vi "SIAM_test_Standalone-ZMQ-Dev.vi"() -> ()   [LabVIEW 2011]
doc: "Tool for TILL ID SIAM hardware test."
uses:
  SIAM_command.ctl
  SIAM-axis.ctl
  Christian/ZeroMQ/Neuer Ordner/File Group 0/vi.lib/addons/zeromq/zmq_socket.lvclass
  Christian/ZeroMQ/Neuer Ordner/File Group 0/vi.lib/addons/zeromq/socket_type.ctl
  Christian/ZeroMQ/Neuer Ordner/File Group 0/vi.lib/addons/zeromq/socket_options.ctl
  Christian/ZeroMQ/Neuer Ordner/File Group 0/vi.lib/addons/zeromq/zmq_context.lvclass
  Christian/ZeroMQ/Neuer Ordner/File Group 0/vi.lib/addons/zeromq/zeromq.lvlib
panel:
  in  "Stop":bool
  in  "recieve socket":refnum<class "zmq_socket.lvclass">
  out "Heartbead":u32
  out "Word1":u32 format="%.0x"
  in  "ScaleConst":T2(array[cluster])=[{"Axis-Ring"=104857665, "Scale"=500.0, "Offset"=1000000.0, "HW min"=0.0, "HW max"=4000.0, "max a"=inf, "max v"=inf, "units"="µm"}, {"Axis-Ring"=102760513, "Scale"=1.0, "Offset"=0.0, "HW min"=-32000.0, "HW max"=32000.0, "max a"=5.0, "max v"=inf, "units"="c"}, {"Axis-Ring"=101711937, "Scale"=1.0, "Offset"=0.0, "HW min"=-32000.0, "HW max"=32000.0, "max a"=0.02, "max v"=inf, "units"="c"}, {"Axis-Ring"=16777217, "Scale"=51200.0, "Offset"=100.0, "HW min"=0.0, "HW max"=5500000.0, "max a"=inf, "max v"=20.0, "units"="mm"}, {"Axis-Ring"=17825793, "Scale"=51200.0, "Offset"=100.0, "HW min"=0.0, "HW max"=3700000.0, "max a"=inf, "max v"=20.0, "units"="mm"}, {"Axis-Ring"=19922945, "Scale"=153600.0, "Offset"=146600.0, "HW min"=0.0, "HW max"=614400.0, "max a"=inf, "max v"=1.0, "units"="Pos"}, {"Axis-Ring"=20971521, "Scale"=25000.1, "Offset"=641.0, "HW min"=0.0, "HW max"=124721.0, "max a"=inf, "max v"=1.0, "units"="Pos"}, {"Axis-Ring"=22020097, "Scale"=1.0, "Offset"=0.0, "HW min"=0.0, "HW max"=51200.0, "max a"=inf, "max v"=inf, "units"="counts"}, {"Axis-Ring"=23068673, "Scale"=10240.0, "Offset"=0.0, "HW min"=0.0, "HW max"=51200.0, "max a"=inf, "max v"=inf, "units"="Pos"}, {"Axis-Ring"=24117249, "Scale"=1.0, "Offset"=0.0, "HW min"=0.0, "HW max"=51200.0, "max a"=inf, "max v"=inf, "units"="counts"}, {"Axis-Ring"=2684354561, "Scale"=1.0, "Offset"=0.0, "HW min"=0.0, "HW max"=65636.0, "max a"=inf, "max v"=inf, "units"="counts"}, {"Axis-Ring"=2685403137, "Scale"=1.0, "Offset"=0.0, "HW min"=0.0, "HW max"=65636.0, "max a"=inf, "max v"=inf, "units"="counts"}, {"Axis-Ring"=2686451713, "Scale"=1.0, "Offset"=0.0, "HW min"=0.0, "HW max"=65636.0, "max a"=inf, "max v"=inf, "units"="counts"}, {"Axis-Ring"=2687500289, "Scale"=1.0, "Offset"=0.0, "HW min"=0.0, "HW max"=65636.0, "max a"=inf, "max v"=inf, "units"="counts"}, {"Axis-Ring"=2688548865, "Scale"=1.0, "Offset"=0.0, "HW min"=0.0, "HW max"=65636.0, "max a"=inf, "max v"=inf, "units"="counts"}, {"Axis-Ring"=2689597441, "Scale"=1.0, "Offset"=1.0, "HW min"=0.0, "HW max"=65636.0, "max a"=inf, "max v"=inf, "units"="counts"}, {"Axis-Ring"=2690646017, "Scale"=1.0, "Offset"=1.0, "HW min"=0.0, "HW max"=65636.0, "max a"=inf, "max v"=inf, "units"="counts"}, {"Axis-Ring"=2691694593, "Scale"=1.0, "Offset"=1.0, "HW min"=0.0, "HW max"=65636.0, "max a"=inf, "max v"=inf, "units"="counts"}, {"Axis-Ring"=2701131777, "Scale"=1.0, "Offset"=1.0, "HW min"=0.0, "HW max"=65636.0, "max a"=inf, "max v"=inf, "units"="counts"}, {"Axis-Ring"=2702180353, "Scale"=1.0, "Offset"=1.0, "HW min"=0.0, "HW max"=65636.0, "max a"=inf, "max v"=inf, "units"="counts"}, {"Axis-Ring"=2703228929, "Scale"=1.0, "Offset"=1.0, "HW min"=0.0, "HW max"=65636.0, "max a"=inf, "max v"=inf, "units"="counts"}, {"Axis-Ring"=2704277505, "Scale"=1.0, "Offset"=1.0, "HW min"=0.0, "HW max"=65636.0, "max a"=inf, "max v"=inf, "units"="counts"}, {"Axis-Ring"=2717908993, "Scale"=1.0, "Offset"=1.0, "HW min"=0.0, "HW max"=65636.0, "max a"=inf, "max v"=inf, "units"="counts"}, {"Axis-Ring"=2718957569, "Scale"=1.0, "Offset"=1.0, "HW min"=0.0, "HW max"=65636.0, "max a"=inf, "max v"=inf, "units"="counts"}, {"Axis-Ring"=2720006145, "Scale"=1.0, "Offset"=1.0, "HW min"=0.0, "HW max"=65636.0, "max a"=inf, "max v"=inf, "units"="counts"}, {"Axis-Ring"=2721054721, "Scale"=1.0, "Offset"=1.0, "HW min"=0.0, "HW max"=65636.0, "max a"=inf, "max v"=inf, "units"="counts"}, {"Axis-Ring"=67108865, "Scale"=1.0, "Offset"=1.0, "HW min"=100000.0, "HW max"=200000.0, "max a"=inf, "max v"=inf, "units"="counts"}, {"Axis-Ring"=68157441, "Scale"=1.0, "Offset"=1.0, "HW min"=100000.0, "HW max"=200000.0, "max a"=inf, "max v"=inf, "units"="counts"}] {"Axis-Ring" items=["255Axis"=16777217, "1-Axis"=17825793, "2-Axis"=18874369, "3-Axis"=19922945, "4-Axis"=20971521, "5-Axis"=22020097, "6-Axis"=23068673, "7-Axis"=24117249, "LED365"=2684354561, "LED385"=2685403137, "LED440"=2686451713, "LED470"=2687500289, "LED510"=2688548865, "LED540"=2689597441, "LED590"=2690646017, "LED640"=2691694593, "DurchR"=2701131777, "DurchG"=2702180353, "DurchB"=2703228929, "AF"=2704277505, "Laser0"=2717908993, "Laser1"=2718957569, "Laser2"=2720006145, "Laser3"=2721054721, "Servo0"=67108865, "Servo1"=68157441, "Servo2"=69206017, "Servo3"=70254593, "0-TMSI"=100663361, "1-TMSI"=101711937, "x-tmsi"=102760513, "y-tmsi"=103809089, "z-tmsi"=104857665, "orca1"=503316481, "orca2"=503316482, "orca3"=503316483, "orca4"=503316484, ""=0]}
  out "Connected":bool
  in  "Format":enum16{"Hex", "dez", "Ascii", "dez16s"}(ring)
  in  "Run":bool
  in  "Clear":bool
  in  "return":string
  in  "Registerkarte":T3(tab)
  in  "Instrument":string(combo)="192.168.99.3 till-x-3"
  in  "connect":bool caption="disconnect"
  out "connect error":errorcluster
  in  "Read":bool
  in  "Axis":T4={"Linear"={"Axis-Ring"=17825793, "Position"=0}, "Linear"={"Axis-Ring"=18874369, "Position"=0}, "Linear 2"={"Axis-Ring"=19922945, "Position"=0}, "Linear 3"={"Axis-Ring"=101711937, "Position"=0}, "Linear"={"Axis-Ring"=102760513, "Position"=0}, "Linear 4"={"Axis-Ring"=2684354561, "Position"=0}, "Linear 5"={"Axis-Ring"=2685403137, "Position"=0}, "Linear 6"={"Axis-Ring"=2687500289, "Position"=0}, "Linear 7"={"Axis-Ring"=2691694593, "Position"=0}, "Linear 8"={"Axis-Ring"=2701131777, "Position"=0}, "Linear 9"={"Axis-Ring"=2717908993, "Position"=0}, "Linear 10"={"Axis-Ring"=2718957569, "Position"=0}, "Linear 11"={"Axis-Ring"=2720006145, "Position"=0}, "Linear 12"={"Axis-Ring"=503316482, "Position"=0}, "Linear 13"={"Axis-Ring"=67108865, "Position"=150000}} {"Linear 13"."Axis-Ring" items=["X-Axis"=16777217, "Y-Axis"=17825793, "Obj"=19922945, "Filter"=20971521, "Trans"=22020097, "FRET"=23068673, "SI"=24117249, "LED365"=2684354561, "LED385"=2685403137, "LED440"=2686451713, "LED470"=2687500289, "LED510"=2688548865, "LED540"=2689597441, "LED590"=2690646017, "LED640"=2691694593, "DurchR"=2701131777, "DurchG"=2702180353, "DurchB"=2703228929, "AF"=2704277505, "Laser0"=2717908993, "Laser1"=2718957569, "Laser2"=2720006145, "Laser3"=2721054721, "Servo0"=67108865, "Servo1"=68157441, "Servo2"=69206017, "Servo3"=70254593]; "Linear 13"."Position" scale=100000.0..200000.0; "Linear 12"."Axis-Ring" items=["255Axis"=16777217, "1-Axis"=17825793, "2-Axis"=18874369, "3-Axis"=19922945, "4-Axis"=20971521, "5-Axis"=22020097, "6-Axis"=23068673, "7-Axis"=24117249, "LED365"=2684354561, "LED385"=2685403137, "LED440"=2686451713, "LED470"=2687500289, "LED510"=2688548865, "LED540"=2689597441, "LED590"=2690646017, "LED640"=2691694593, "DurchR"=2701131777, "DurchG"=2702180353, "DurchB"=2703228929, "AF"=2704277505, "Laser0"=2717908993, "Laser1"=2718957569, "Laser2"=2720006145, "Laser3"=2721054721, "Servo0"=67108865, "Servo1"=68157441, "Servo2"=69206017, "Servo3"=70254593, "0-TMSI"=100663361, "1-TMSI"=101711937, "x-tmsi"=102760513, "y-tmsi"=103809089, "z-tmsi"=104857665, "orca1"=503316481, "orca2"=503316482, "orca3"=503316483, "orca4"=503316484, ""=0]; "Linear 12"."Position" scale=0.0..100.0; "Linear 11"."Axis-Ring" items=["255Axis"=16777217, "1-Axis"=17825793, "2-Axis"=18874369, "3-Axis"=19922945, "4-Axis"=20971521, "5-Axis"=22020097, "6-Axis"=23068673, "7-Axis"=24117249, "LED365"=2684354561, "LED385"=2685403137, "LED440"=2686451713, "LED470"=2687500289, "LED510"=2688548865, "LED540"=2689597441, "LED590"=2690646017, "LED640"=2691694593, "DurchR"=2701131777, "DurchG"=2702180353, "DurchB"=2703228929, "AF"=2704277505, "Laser0"=2717908993, "Laser1"=2718957569, "Laser2"=2720006145, "Laser3"=2721054721, "Servo0"=67108865, "Servo1"=68157441, "Servo2"=69206017, "Servo3"=70254593, "0-TMSI"=100663361, "1-TMSI"=101711937, "x-tmsi"=102760513, "y-tmsi"=103809089, "z-tmsi"=104857665, "orca1"=503316481, "orca2"=503316482, "orca3"=503316483, "orca4"=503316484, ""=0]; "Linear 11"."Position" scale=0.0..65000.0; "Linear 10"."Axis-Ring" items=["255Axis"=16777217, "1-Axis"=17825793, "2-Axis"=18874369, "3-Axis"=19922945, "4-Axis"=20971521, "5-Axis"=22020097, "6-Axis"=23068673, "7-Axis"=24117249, "LED365"=2684354561, "LED385"=2685403137, "LED440"=2686451713, "LED470"=2687500289, "LED510"=2688548865, "LED540"=2689597441, "LED590"=2690646017, "LED640"=2691694593, "DurchR"=2701131777, "DurchG"=2702180353, "DurchB"=2703228929, "AF"=2704277505, "Laser0"=2717908993, "Laser1"=2718957569, "Laser2"=2720006145, "Laser3"=2721054721, "Servo0"=67108865, "Servo1"=68157441, "Servo2"=69206017, "Servo3"=70254593, "0-TMSI"=100663361, "1-TMSI"=101711937, "x-tmsi"=102760513, "y-tmsi"=103809089, "z-tmsi"=104857665, "orca1"=503316481, "orca2"=503316482, "orca3"=503316483, "orca4"=503316484, ""=0]; "Linear 10"."Position" scale=0.0..65000.0; "Linear 9"."Axis-Ring" items=["255Axis"=16777217, "1-Axis"=17825793, "2-Axis"=18874369, "3-Axis"=19922945, "4-Axis"=20971521, "5-Axis"=22020097, "6-Axis"=23068673, "7-Axis"=24117249, "LED365"=2684354561, "LED385"=2685403137, "LED440"=2686451713, "LED470"=2687500289, "LED510"=2688548865, "LED540"=2689597441, "LED590"=2690646017, "LED640"=2691694593, "DurchR"=2701131777, "DurchG"=2702180353, "DurchB"=2703228929, "AF"=2704277505, "Laser0"=2717908993, "Laser1"=2718957569, "Laser2"=2720006145, "Laser3"=2721054721, "Servo0"=67108865, "Servo1"=68157441, "Servo2"=69206017, "Servo3"=70254593, "0-TMSI"=100663361, "1-TMSI"=101711937, "x-tmsi"=102760513, "y-tmsi"=103809089, "z-tmsi"=104857665, "orca1"=503316481, "orca2"=503316482, "orca3"=503316483, "orca4"=503316484, ""=0]; "Linear 9"."Position" scale=0.0..65000.0; "Linear 8"."Axis-Ring" items=["255Axis"=16777217, "1-Axis"=17825793, "2-Axis"=18874369, "3-Axis"=19922945, "4-Axis"=20971521, "5-Axis"=22020097, "6-Axis"=23068673, "7-Axis"=24117249, "LED365"=2684354561, "LED385"=2685403137, "LED440"=2686451713, "LED470"=2687500289, "LED510"=2688548865, "LED540"=2689597441, "LED590"=2690646017, "LED640"=2691694593, "DurchR"=2701131777, "DurchG"=2702180353, "DurchB"=2703228929, "AF"=2704277505, "Laser0"=2717908993, "Laser1"=2718957569, "Laser2"=2720006145, "Laser3"=2721054721, "Servo0"=67108865, "Servo1"=68157441, "Servo2"=69206017, "Servo3"=70254593, "0-TMSI"=100663361, "1-TMSI"=101711937, "x-tmsi"=102760513, "y-tmsi"=103809089, "z-tmsi"=104857665, "orca1"=503316481, "orca2"=503316482, "orca3"=503316483, "orca4"=503316484, ""=0]; "Linear 8"."Position" scale=0.0..65000.0; "Linear 7"."Axis-Ring" items=["255Axis"=16777217, "1-Axis"=17825793, "2-Axis"=18874369, "3-Axis"=19922945, "4-Axis"=20971521, "5-Axis"=22020097, "6-Axis"=23068673, "7-Axis"=24117249, "LED365"=2684354561, "LED385"=2685403137, "LED440"=2686451713, "LED470"=2687500289, "LED510"=2688548865, "LED540"=2689597441, "LED590"=2690646017, "LED640"=2691694593, "DurchR"=2701131777, "DurchG"=2702180353, "DurchB"=2703228929, "AF"=2704277505, "Laser0"=2717908993, "Laser1"=2718957569, "Laser2"=2720006145, "Laser3"=2721054721, "Servo0"=67108865, "Servo1"=68157441, "Servo2"=69206017, "Servo3"=70254593, "0-TMSI"=100663361, "1-TMSI"=101711937, "x-tmsi"=102760513, "y-tmsi"=103809089, "z-tmsi"=104857665, "orca1"=503316481, "orca2"=503316482, "orca3"=503316483, "orca4"=503316484, ""=0]; "Linear 7"."Position" scale=0.0..65000.0; "Linear 6"."Axis-Ring" items=["255Axis"=16777217, "1-Axis"=17825793, "2-Axis"=18874369, "3-Axis"=19922945, "4-Axis"=20971521, "5-Axis"=22020097, "6-Axis"=23068673, "7-Axis"=24117249, "LED365"=2684354561, "LED385"=2685403137, "LED440"=2686451713, "LED470"=2687500289, "LED510"=2688548865, "LED540"=2689597441, "LED590"=2690646017, "LED640"=2691694593, "DurchR"=2701131777, "DurchG"=2702180353, "DurchB"=2703228929, "AF"=2704277505, "Laser0"=2717908993, "Laser1"=2718957569, "Laser2"=2720006145, "Laser3"=2721054721, "Servo0"=67108865, "Servo1"=68157441, "Servo2"=69206017, "Servo3"=70254593, "0-TMSI"=100663361, "1-TMSI"=101711937, "x-tmsi"=102760513, "y-tmsi"=103809089, "z-tmsi"=104857665, "orca1"=503316481, "orca2"=503316482, "orca3"=503316483, "orca4"=503316484, ""=0]; "Linear 6"."Position" scale=0.0..65000.0; "Linear 5"."Axis-Ring" items=["255Axis"=16777217, "1-Axis"=17825793, "2-Axis"=18874369, "3-Axis"=19922945, "4-Axis"=20971521, "5-Axis"=22020097, "6-Axis"=23068673, "7-Axis"=24117249, "LED365"=2684354561, "LED385"=2685403137, "LED440"=2686451713, "LED470"=2687500289, "LED510"=2688548865, "LED540"=2689597441, "LED590"=2690646017, "LED640"=2691694593, "DurchR"=2701131777, "DurchG"=2702180353, "DurchB"=2703228929, "AF"=2704277505, "Laser0"=2717908993, "Laser1"=2718957569, "Laser2"=2720006145, "Laser3"=2721054721, "Servo0"=67108865, "Servo1"=68157441, "Servo2"=69206017, "Servo3"=70254593, "0-TMSI"=100663361, "1-TMSI"=101711937, "x-tmsi"=102760513, "y-tmsi"=103809089, "z-tmsi"=104857665, "orca1"=503316481, "orca2"=503316482, "orca3"=503316483, "orca4"=503316484, ""=0]; "Linear 5"."Position" scale=0.0..65000.0; "Linear 4"."Axis-Ring" items=["255Axis"=16777217, "1-Axis"=17825793, "2-Axis"=18874369, "3-Axis"=19922945, "4-Axis"=20971521, "5-Axis"=22020097, "6-Axis"=23068673, "7-Axis"=24117249, "LED365"=2684354561, "LED385"=2685403137, "LED440"=2686451713, "LED470"=2687500289, "LED510"=2688548865, "LED540"=2689597441, "LED590"=2690646017, "LED640"=2691694593, "DurchR"=2701131777, "DurchG"=2702180353, "DurchB"=2703228929, "AF"=2704277505, "Laser0"=2717908993, "Laser1"=2718957569, "Laser2"=2720006145, "Laser3"=2721054721, "Servo0"=67108865, "Servo1"=68157441, "Servo2"=69206017, "Servo3"=70254593, "0-TMSI"=100663361, "1-TMSI"=101711937, "x-tmsi"=102760513, "y-tmsi"=103809089, "z-tmsi"=104857665, "orca1"=503316481, "orca2"=503316482, "orca3"=503316483, "orca4"=503316484, ""=0]; "Linear 4"."Position" scale=0.0..65000.0; "Linear"."Axis-Ring" items=["255Axis"=16777217, "1-Axis"=17825793, "2-Axis"=18874369, "3-Axis"=19922945, "4-Axis"=20971521, "5-Axis"=22020097, "6-Axis"=23068673, "7-Axis"=24117249, "LED365"=2684354561, "LED385"=2685403137, "LED440"=2686451713, "LED470"=2687500289, "LED510"=2688548865, "LED540"=2689597441, "LED590"=2690646017, "LED640"=2691694593, "DurchR"=2701131777, "DurchG"=2702180353, "DurchB"=2703228929, "AF"=2704277505, "Laser0"=2717908993, "Laser1"=2718957569, "Laser2"=2720006145, "Laser3"=2721054721, "Servo0"=67108865, "Servo1"=68157441, "Servo2"=69206017, "Servo3"=70254593, "0-TMSI"=100663361, "1-TMSI"=101711937, "x-tmsi"=102760513, "y-tmsi"=103809089, "z-tmsi"=104857665, "orca1"=503316481, "orca2"=503316482, "orca3"=503316483, "orca4"=503316484, ""=0]; "Linear"."Position" scale=-32000.0..32000.0; "Linear 3"."Axis-Ring" items=["255Axis"=16777217, "1-Axis"=17825793, "2-Axis"=18874369, "3-Axis"=19922945, "4-Axis"=20971521, "5-Axis"=22020097, "6-Axis"=23068673, "7-Axis"=24117249, "LED365"=2684354561, "LED385"=2685403137, "LED440"=2686451713, "LED470"=2687500289, "LED510"=2688548865, "LED540"=2689597441, "LED590"=2690646017, "LED640"=2691694593, "DurchR"=2701131777, "DurchG"=2702180353, "DurchB"=2703228929, "AF"=2704277505, "Laser0"=2717908993, "Laser1"=2718957569, "Laser2"=2720006145, "Laser3"=2721054721, "Servo0"=67108865, "Servo1"=68157441, "Servo2"=69206017, "Servo3"=70254593, "0-TMSI"=100663361, "1-TMSI"=101711937, "x-tmsi"=102760513, "y-tmsi"=103809089, "z-tmsi"=104857665, "orca1"=503316481, "orca2"=503316482, "orca3"=503316483, "orca4"=503316484, ""=0]; "Linear 3"."Position" scale=-32000.0..32000.0; "Linear 2"."Axis-Ring" items=["255Axis"=16777217, "1-Axis"=17825793, "2-Axis"=18874369, "3-Axis"=19922945, "4-Axis"=20971521, "5-Axis"=22020097, "6-Axis"=23068673, "7-Axis"=24117249, "LED365"=2684354561, "LED385"=2685403137, "LED440"=2686451713, "LED470"=2687500289, "LED510"=2688548865, "LED540"=2689597441, "LED590"=2690646017, "LED640"=2691694593, "DurchR"=2701131777, "DurchG"=2702180353, "DurchB"=2703228929, "AF"=2704277505, "Laser0"=2717908993, "Laser1"=2718957569, "Laser2"=2720006145, "Laser3"=2721054721, "Servo0"=67108865, "Servo1"=68157441, "Servo2"=69206017, "Servo3"=70254593, "0-TMSI"=100663361, "1-TMSI"=101711937, "x-tmsi"=102760513, "y-tmsi"=103809089, "z-tmsi"=104857665, "orca1"=503316481, "orca2"=503316482, "orca3"=503316483, "orca4"=503316484, ""=0]; "Linear 2"."Position" scale=-100000.0..50000.0; "Linear"."Axis-Ring" items=["255Axis"=16777217, "1-Axis"=17825793, "2-Axis"=18874369, "3-Axis"=19922945, "4-Axis"=20971521, "5-Axis"=22020097, "6-Axis"=23068673, "7-Axis"=24117249, "LED365"=2684354561, "LED385"=2685403137, "LED440"=2686451713, "LED470"=2687500289, "LED510"=2688548865, "LED540"=2689597441, "LED590"=2690646017, "LED640"=2691694593, "DurchR"=2701131777, "DurchG"=2702180353, "DurchB"=2703228929, "AF"=2704277505, "Laser0"=2717908993, "Laser1"=2718957569, "Laser2"=2720006145, "Laser3"=2721054721, "Servo0"=67108865, "Servo1"=68157441, "Servo2"=69206017, "Servo3"=70254593, "0-TMSI"=100663361, "1-TMSI"=101711937, "x-tmsi"=102760513, "y-tmsi"=103809089, "z-tmsi"=104857665, "orca1"=503316481, "orca2"=503316482, "orca3"=503316483, "orca4"=503316484, ""=0]; "Linear"."Position" scale=-250000.0..250000.0; "Linear"."Axis-Ring" items=["255Axis"=16777217, "1-Axis"=17825793, "2-Axis"=18874369, "3-Axis"=19922945, "4-Axis"=20971521, "5-Axis"=22020097, "6-Axis"=23068673, "7-Axis"=24117249, "LED365"=2684354561, "LED385"=2685403137, "LED440"=2686451713, "LED470"=2687500289, "LED510"=2688548865, "LED540"=2689597441, "LED590"=2690646017, "LED640"=2691694593, "DurchR"=2701131777, "DurchG"=2702180353, "DurchB"=2703228929, "AF"=2704277505, "Laser0"=2717908993, "Laser1"=2718957569, "Laser2"=2720006145, "Laser3"=2721054721, "Servo0"=67108865, "Servo1"=68157441, "Servo2"=69206017, "Servo3"=70254593, "0-TMSI"=100663361, "1-TMSI"=101711937, "x-tmsi"=102760513, "y-tmsi"=103809089, "z-tmsi"=104857665, "orca1"=503316481, "orca2"=503316482, "orca3"=503316483, "orca4"=503316484, ""=0]; "Linear"."Position" scale=-1024000.0..1024000.0}
  in  "Array":T5(array[cluster])=[{"Digital-out"=enum."cam1", "Boolean"=FALSE}, {"Digital-out"=enum."cam2", "Boolean"=FALSE}, {"Digital-out"=enum."led2", "Boolean"=FALSE}, {"Digital-out"=enum."led3", "Boolean"=FALSE}, {"Digital-out"=enum."led4", "Boolean"=FALSE}, {"Digital-out"=enum."led5", "Boolean"=FALSE}, {"Digital-out"=enum."led5", "Boolean"=FALSE}, {"Digital-out"=enum."led7", "Boolean"=FALSE}, {"Digital-out"=enum."led8", "Boolean"=FALSE}, {"Digital-out"=enum."durchR", "Boolean"=FALSE}, {"Digital-out"=enum."tsm-pwr", "Boolean"=FALSE}, {"Digital-out"=enum."dc-pwr", "Boolean"=FALSE}, {"Digital-out"=enum."laser-pwr", "Boolean"=FALSE}, {"Digital-out"=enum."Laser0", "Boolean"=FALSE}, {"Digital-out"=enum."Laser1", "Boolean"=FALSE}, {"Digital-out"=enum."Laser2", "Boolean"=FALSE}, {"Digital-out"=enum."Laser3", "Boolean"=FALSE}, {"Digital-out"=enum."TrigOut", "Boolean"=FALSE}, {"Digital-out"=enum."SMB1", "Boolean"=FALSE}]
  in  "xy":T6
  in  "step":i32=42345
  in  "Calculate SIM":bool
  out "Camera":T7={"Camera-Expos ms"=0.0, "CameraImages"=7, "cam fps min."=0.0}
  in  "Constants":T9={"galvox-Line0"=14814, "GalvoX-Blanking"=15000.0, "galvox-count/pix"=-2.474, "Camera-StartLine"=-62, "Camera-Endline"=4000, "Wobbel-total"=4280.0, "SM_ticks"=20, "Trigger_ticks"=38, "galvoxAccel"=5.0, "WobbelAccel"=0.01, "zAccel"=0.05, "z-delay-ticks"=700, "SCMOS-LineSpeed [10µs]"=1.25, "RS height- Pix"=100, "extra-xgalvo"=83.0, "zcommand"=4026531840, "min turn ticks"=500.0} {"zcommand" format="%x" items=["end_no_ticket"=4027514895, "end_ticket"=4027518991, "NoOp"=4026531840, "Read ticks"=4026535936, "Read ticks to var"=4026535938, "Read IP"=4043313152, "Read IP into var"=4043313154, "Set IP from var"=4043309059, "Set IP from var, relative"=4043313155, "branchRel_if_equal"=4043374849, "decrement_branchRel_if_equal"=4043374945, "decrement_branchRel_if_greaterequal"=4043375201, "decrement_branchRel_if_greaterequal_withTicket"=4043379297, "decrement_branchRel_if_smaller"=4043375457, "increment_branchRel_if_smaller"=4043375473, "readVar"=4060090368, "writeVar"=4060086273, "copyVar0_from_var1"=4060086275, "math_addToVariable"=4076863488, "math_addVToVariable"=4076863489, "math_subToVariable"=4076863490, "math_subVToVariable"=4076863491, "math_multToVariable"=4076863492, "math_multvToVariable"=4076863493, "math_divideToVariable"=4076863494, "math_divideVToVariable"=4076863495, "math_modToVariable"=4076863496, "math_modVToVariable"=4076863497, "logic_and"=4093640704, "logic_or"=4093640706, "logic_xor"=4093640708, "bitshift"=4093640712, "I2C-write"=335544337, "I2C-read"=335548433, "Cam-SPI-write"=3254779905, "UART0-VC-Baud-write"=469958673, "UART0-VC-Baud-read"=469962768, "UART0-VC-write"=469762065, "UART0-VC-write-Var"=469762067, "UART0-VC-read-availabe-bytes-to-var"=470355970, "UART0-VC-read-availabe-bytes"=470355984, "UART0-VC-read-skip-bytes"=469831681, "UART0-VC-read"=469766160, "UART0-VC-read-Var"=469766162, "UART1-TSM-Baud-write"=486735889, "UART1-TSM-Baud-read"=486739984, "UART1-TSM-write"=486539281, "UART1-TSM-write-Var"=486539283, "UART1-TSM-read-availabe-bytes-to-var"=487133186, "UART1-TSM-read-availabe-bytes"=487133200, "UART1-TSM-read-skip-bytes"=486604801, "UART1-TSM-read-skip-bytes"=486608897, "UART1-TSM-read"=486543376, "UART1-TSM-read-Var"=486543378, "UART2-Laser-Baud-write"=503513105, "UART2-Baud-read"=503517200, "UART2-write"=503316497, "UART2-write-Var"=503316499, "UART2-read-availabe-bytes-to-var"=503910402, "UART2-read-availabe-bytes"=503910416, "UART2-read-skip-bytes"=503386113, "UART2-read"=503320592, "UART2-read-Var"=503320594, "UART3-Baud-write"=520290321, "UART3-Baud-read"=520294416, "UART3-write"=520093713, "UART3-write-Var"=520093715, "UART3-read-availabe-bytes-to-var"=520687618, "UART3-read-availabe-bytes"=520687632, "UART3-read-skip-bytes"=520163329, "UART3-read"=520097808, "UART3-read-Var"=520097810, "IO-read_bank0"=3489665024, "IO-write_bank0"=3489660929, "IO-read_bank1"=3506442240, "IO-write_bank1"=3506438145, "DA0-0_LED365"=2684354561, "DA0-1_LED385"=2685403137, "DA0-2_LED440"=2686451713, "DA0-3_LED470"=2687500289, "DA0-4_LED510"=2688548865, "DA0-5_LED550"=2689597441, "DA0-6_LED590"=2690646017, "DA0-7_LED640"=2691694593, "DA1-0_LED-R"=2701131777, "DA1-1_LED-G"=2702180353, "DA1-2_LED-B"=2703228929, "DA1-3_LED-AF"=2704277505, "DA1-4"=2705326081, "DA1-5"=2706374657, "DA1-6"=2707423233, "DA1-7"=2708471809, "DA2-Laser0"=2717908993, "DA2-Laser1"=2718957569, "DA2-Laser2"=2720006145, "DA2-Laser3"=2721054721, "DA2-Laser4"=2722103297, "Analog-read_AD0-0"=2818576384, "Analog-read-store_AD0-0"=2818572290, "AF-Register-transfer r/w"=2835349505, "AF-Register-read"=2835353600, "AF-Register-read-to-var"=2835353602, "AF-Transfer-from-var"=2835349507, "IO-delay_bank0"=3489923073, "IO-delay_bank0_fromVar"=3489923075, "read_cam_clock"=3289124864, "store_cam_clock"=3289120770, "read_cam_phase"=3289190400, "store_cam_phase"=3289186306, "store_cam_phase-t"=3289190402, "r_cam1_NHS"=3254980608, "w_cam1_NHS"=3254976513, "r_cam1_NVS"=3255046144, "w_cam1_NVS"=3255042049, "r_cam1_npx"=3255111680, "w_cam1_npx"=3255107585, "r_cam1_npy"=3255177216, "w_cam1_npy"=3255173121, "r_cam1_xhswait"=3255439360, "w_cam1_xhswait"=3255435265, "r_cam1_xvs_wait"=3255504896, "w_cam1_xvs_wait"=3255500801, "r_cam1_framcounter"=3255570432, "r_cam1_line"=3255635968, "r_cam1_xhs-counter"=3255701504, "r_cam2_NHS"=3271757824, "w_cam2_NHS"=3271753729, "r_cam2_NVS"=3271823360, "w_cam2_NVS"=3271819265, "r_cam2_npx"=3271888896, "w_cam2_npx"=3271884801, "r_cam2_npy"=3271954432, "w_cam2_npy"=3271950337, "r_cam2_xvs_wait"=3272282112, "w_cam2_xvs_wait"=3272278017, "r_cam2_framcounter"=3272347648, "r_cam2_line"=3272413184, "r_cam2_xhs-counter"=3272478720, "start TMSI"=102694919, "set_1Galvo"=101712113, "set_x-Galvo"=102760689, "set_y-Galvo"=103809265, "set_z-Fokus"=104857841, "set_1Galvo_position-only"=101711937, "set_x-Galvo_position-only"=102760513, "set_y-Galvo_position-only"=103809089, "set_z-Fokus_position-only"=104857665, "set_x-Galvo_position-only_ticket"=102764609, "set_y-Galvo_position-only_ticket"=103813185, "set_z-Fokus_position-only_ticket"=104861761, "set_1Galvo_relativ-only"=101712001, "set_x-Galvo_relativ-only"=102760577, "set_y-Galvo_relativ-only"=103809153, "set_z-Fokus_relativ-only"=104857729, "set_1Galvo_speed-only"=101711905, "set_x-Galvo_speed-only"=102760481, "set_y-Galvo_speed-only"=103809057, "set_z-Fokus_speed-only"=104857633, "set_1Galvo_acc-only"=101711889, "set_x-Galvo_acc-only"=102760465, "set_y-Galvo_acc-only"=103809041, "set_z-Fokus_acc-only"=104857617, "read_1Galvo_ticket"=101716032, "read_x-Galvo_ticket"=102764608, "read_y-Galvo_ticket"=103813184, "read_z-Focus_ticket"=104861760, "x-Galvo_pos_fromVar"=102760515, "y-Galvo_pos_fromVar"=103809091, "z-Focus_pos_fromVar"=104857667, "Servo0"=67108865, "Servo0-enable"=68091911, "Servo0-disable"=68091919, "Servo1"=68157441, "Servo1-enable"=69140487, "Servo1-disable"=69140495, "Servo2-enable"=70189063, "Servo2"=69206017, "Servo3-enable"=71237639, "Servo3"=70254593, "x-ssi-init"=202309639, "x-ssi-disable"=202309647, "x-ssi-Bits"=201523201, "x-ssi-Read"=201330688, "x-ssi-ReadToVar"=201326594, "x-ssi-ReadToVar-ticket"=201330690, "y-ssi-init"=203358215, "y-ssi-disable"=203358223, "y-ssi-Bits"=202571777, "y-ssi-Read"=202379264, "y-ssi-ReadToVar"=202375170, "y-ssi-ReadToVat-ticket"=202379266]; "SCMOS-LineSpeed [10µs]" format="%#.6f" items=["EdgeFast-285MHz"=0.9175, "EdgeSlow-95MHz"=2.7525, "Panda4.2"=2.7766, "sensocam183"=1.2, "mer2000-12"=2.4996, "mer2000-8bit"=1.25]; "galvox-count/pix" format="%#_5f"}
  in  "User":T10={"z-distance_motorunits"=100, "#planes"=1, "Digital-out"=enum."Laser1", "NoOfPhaseImages"=7} {"#planes" min=1}
  in  "SendScript":bool
  in  "Load":bool
  in  "Save":bool
  in  "ClearScript":bool
  in  "Script":T11(array[cluster])=[{"Delay 10µs"=0, "command"=4027514895, "P0"=0, "P1"=0, "P2"=0, "P3"=0, "P4"=0, "P5-ticket"=0, "comment"=""}] {"command" format="%x" items=["end_no_ticket"=4027514895, "end_ticket"=4027518991, "NoOp"=4026531840, "Read ticks"=4026535936, "Read ticks to var"=4026535938, "Read IP"=4043313152, "Read IP into var"=4043313154, "Set IP from var"=4043309059, "Set IP from var, relative"=4043313155, "branchRel_if_equal"=4043374849, "decrement_branchRel_if_equal"=4043374945, "decrement_branchRel_if_greaterequal"=4043375201, "decrement_branchRel_if_greaterequal_withTicket"=4043379297, "decrement_branchRel_if_smaller"=4043375457, "increment_branchRel_if_smaller"=4043375473, "readVar"=4060090368, "writeVar"=4060086273, "copyVar0_from_var1"=4060086275, "math_addToVariable"=4076863488, "math_addVToVariable"=4076863489, "math_subToVariable"=4076863490, "math_subVToVariable"=4076863491, "math_multToVariable"=4076863492, "math_multvToVariable"=4076863493, "math_divideToVariable"=4076863494, "math_divideVToVariable"=4076863495, "math_modToVariable"=4076863496, "math_modVToVariable"=4076863497, "logic_and"=4093640704, "logic_or"=4093640706, "logic_xor"=4093640708, "bitshift"=4093640712, "I2C-write"=335544337, "I2C-read"=335548433, "Cam-SPI-write"=3254779905, "UART0-VC-Baud-write"=469958673, "UART0-VC-Baud-read"=469962768, "UART0-VC-write"=469762065, "UART0-VC-write-Var"=469762067, "UART0-VC-read-availabe-bytes-to-var"=470355970, "UART0-VC-read-availabe-bytes"=470355984, "UART0-VC-read-skip-bytes"=469831681, "UART0-VC-read"=469766160, "UART0-VC-read-Var"=469766162, "UART1-TSM-Baud-write"=486735889, "UART1-TSM-Baud-read"=486739984, "UART1-TSM-write"=486539281, "UART1-TSM-write-Var"=486539283, "UART1-TSM-read-availabe-bytes-to-var"=487133186, "UART1-TSM-read-availabe-bytes"=487133200, "UART1-TSM-read-skip-bytes"=486604801, "UART1-TSM-read-skip-bytes"=486608897, "UART1-TSM-read"=486543376, "UART1-TSM-read-Var"=486543378, "UART2-Laser-Baud-write"=503513105, "UART2-Baud-read"=503517200, "UART2-write"=503316497, "UART2-write-Var"=503316499, "UART2-read-availabe-bytes-to-var"=503910402, "UART2-read-availabe-bytes"=503910416, "UART2-read-skip-bytes"=503386113, "UART2-read"=503320592, "UART2-read-Var"=503320594, "UART3-Baud-write"=520290321, "UART3-Baud-read"=520294416, "UART3-write"=520093713, "UART3-write-Var"=520093715, "UART3-read-availabe-bytes-to-var"=520687618, "UART3-read-availabe-bytes"=520687632, "UART3-read-skip-bytes"=520163329, "UART3-read"=520097808, "UART3-read-Var"=520097810, "IO-read_bank0"=3489665024, "IO-write_bank0"=3489660929, "IO-read_bank1"=3506442240, "IO-write_bank1"=3506438145, "DA0-0_LED365"=2684354561, "DA0-1_LED385"=2685403137, "DA0-2_LED440"=2686451713, "DA0-3_LED470"=2687500289, "DA0-4_LED510"=2688548865, "DA0-5_LED550"=2689597441, "DA0-6_LED590"=2690646017, "DA0-7_LED640"=2691694593, "DA1-0_LED-R"=2701131777, "DA1-1_LED-G"=2702180353, "DA1-2_LED-B"=2703228929, "DA1-3_LED-AF"=2704277505, "DA1-4"=2705326081, "DA1-5"=2706374657, "DA1-6"=2707423233, "DA1-7"=2708471809, "DA2-Laser0"=2717908993, "DA2-Laser1"=2718957569, "DA2-Laser2"=2720006145, "DA2-Laser3"=2721054721, "DA2-Laser4"=2722103297, "Analog-read_AD0-0"=2818576384, "Analog-read-store_AD0-0"=2818572290, "AF-Register-transfer r/w"=2835349505, "AF-Register-read"=2835353600, "AF-Register-read-to-var"=2835353602, "AF-Transfer-from-var"=2835349507, "IO-delay_bank0"=3489923073, "IO-delay_bank0_fromVar"=3489923075, "read_cam_clock"=3289124864, "store_cam_clock"=3289120770, "read_cam_phase"=3289190400, "store_cam_phase"=3289186306, "store_cam_phase-t"=3289190402, "r_cam1_NHS"=3254980608, "w_cam1_NHS"=3254976513, "r_cam1_NVS"=3255046144, "w_cam1_NVS"=3255042049, "r_cam1_npx"=3255111680, "w_cam1_npx"=3255107585, "r_cam1_npy"=3255177216, "w_cam1_npy"=3255173121, "r_cam1_xhswait"=3255439360, "w_cam1_xhswait"=3255435265, "r_cam1_xvs_wait"=3255504896, "w_cam1_xvs_wait"=3255500801, "r_cam1_framcounter"=3255570432, "r_cam1_line"=3255635968, "r_cam1_xhs-counter"=3255701504, "r_cam2_NHS"=3271757824, "w_cam2_NHS"=3271753729, "r_cam2_NVS"=3271823360, "w_cam2_NVS"=3271819265, "r_cam2_npx"=3271888896, "w_cam2_npx"=3271884801, "r_cam2_npy"=3271954432, "w_cam2_npy"=3271950337, "r_cam2_xvs_wait"=3272282112, "w_cam2_xvs_wait"=3272278017, "r_cam2_framcounter"=3272347648, "r_cam2_line"=3272413184, "r_cam2_xhs-counter"=3272478720, "start TMSI"=102694919, "set_1Galvo"=101712113, "set_x-Galvo"=102760689, "set_y-Galvo"=103809265, "set_z-Fokus"=104857841, "set_1Galvo_position-only"=101711937, "set_x-Galvo_position-only"=102760513, "set_y-Galvo_position-only"=103809089, "set_z-Fokus_position-only"=104857665, "set_x-Galvo_position-only_ticket"=102764609, "set_y-Galvo_position-only_ticket"=103813185, "set_z-Fokus_position-only_ticket"=104861761, "set_1Galvo_relativ-only"=101712001, "set_x-Galvo_relativ-only"=102760577, "set_y-Galvo_relativ-only"=103809153, "set_z-Fokus_relativ-only"=104857729, "set_1Galvo_speed-only"=101711905, "set_x-Galvo_speed-only"=102760481, "set_y-Galvo_speed-only"=103809057, "set_z-Fokus_speed-only"=104857633, "set_1Galvo_acc-only"=101711889, "set_x-Galvo_acc-only"=102760465, "set_y-Galvo_acc-only"=103809041, "set_z-Fokus_acc-only"=104857617, "read_1Galvo_ticket"=101716032, "read_x-Galvo_ticket"=102764608, "read_y-Galvo_ticket"=103813184, "read_z-Focus_ticket"=104861760, "x-Galvo_pos_fromVar"=102760515, "y-Galvo_pos_fromVar"=103809091, "z-Focus_pos_fromVar"=104857667, "Servo0"=67108865, "Servo0-enable"=68091911, "Servo0-disable"=68091919, "Servo1"=68157441, "Servo1-enable"=69140487, "Servo1-disable"=69140495, "Servo2-enable"=70189063, "Servo2"=69206017, "Servo3-enable"=71237639, "Servo3"=70254593, "x-ssi-init"=202309639, "x-ssi-disable"=202309647, "x-ssi-Bits"=201523201, "x-ssi-Read"=201330688, "x-ssi-ReadToVar"=201326594, "x-ssi-ReadToVar-ticket"=201330690, "y-ssi-init"=203358215, "y-ssi-disable"=203358223, "y-ssi-Bits"=202571777, "y-ssi-Read"=202379264, "y-ssi-ReadToVar"=202375170, "y-ssi-ReadToVat-ticket"=202379266]; "P5-ticket" format="%.0x"; "P0" format="%.0x"; "P1" format="%.0x"}
  in  "Clear direct":bool
  in  "UART: 0..3":u8=2 max=3
  in  "Uart-TSM":bool
  in  "Uart-Ascii":bool
  in  "Special":bool
  in  "direkt command queue":T11(array[cluster])=[{"Delay 10µs"=0, "command"=102694919, "P0"=0, "P1"=0, "P2"=0, "P3"=0, "P4"=0, "P5-ticket"=0, "comment"=""}] {"command" format="%x" items=["end_no_ticket"=4027514895, "end_ticket"=4027518991, "NoOp"=4026531840, "Read ticks"=4026535936, "Read ticks to var"=4026535938, "Read IP"=4043313152, "Read IP into var"=4043313154, "Set IP from var"=4043309059, "Set IP from var, relative"=4043313155, "branchRel_if_equal"=4043374849, "decrement_branchRel_if_equal"=4043374945, "decrement_branchRel_if_greaterequal"=4043375201, "decrement_branchRel_if_greaterequal_withTicket"=4043379297, "decrement_branchRel_if_smaller"=4043375457, "increment_branchRel_if_smaller"=4043375473, "readVar"=4060090368, "writeVar"=4060086273, "copyVar0_from_var1"=4060086275, "math_addToVariable"=4076863488, "math_addVToVariable"=4076863489, "math_subToVariable"=4076863490, "math_subVToVariable"=4076863491, "math_multToVariable"=4076863492, "math_multvToVariable"=4076863493, "math_divideToVariable"=4076863494, "math_divideVToVariable"=4076863495, "math_modToVariable"=4076863496, "math_modVToVariable"=4076863497, "logic_and"=4093640704, "logic_or"=4093640706, "logic_xor"=4093640708, "bitshift"=4093640712, "I2C-write"=335544337, "I2C-read"=335548433, "Cam-SPI-write"=3254779905, "UART0-VC-Baud-write"=469958673, "UART0-VC-Baud-read"=469962768, "UART0-VC-write"=469762065, "UART0-VC-write-Var"=469762067, "UART0-VC-read-availabe-bytes-to-var"=470355970, "UART0-VC-read-availabe-bytes"=470355984, "UART0-VC-read-skip-bytes"=469831681, "UART0-VC-read"=469766160, "UART0-VC-read-Var"=469766162, "UART1-TSM-Baud-write"=486735889, "UART1-TSM-Baud-read"=486739984, "UART1-TSM-write"=486539281, "UART1-TSM-write-Var"=486539283, "UART1-TSM-read-availabe-bytes-to-var"=487133186, "UART1-TSM-read-availabe-bytes"=487133200, "UART1-TSM-read-skip-bytes"=486604801, "UART1-TSM-read-skip-bytes"=486608897, "UART1-TSM-read"=486543376, "UART1-TSM-read-Var"=486543378, "UART2-Laser-Baud-write"=503513105, "UART2-Baud-read"=503517200, "UART2-write"=503316497, "UART2-write-Var"=503316499, "UART2-read-availabe-bytes-to-var"=503910402, "UART2-read-availabe-bytes"=503910416, "UART2-read-skip-bytes"=503386113, "UART2-read"=503320592, "UART2-read-Var"=503320594, "UART3-Baud-write"=520290321, "UART3-Baud-read"=520294416, "UART3-write"=520093713, "UART3-write-Var"=520093715, "UART3-read-availabe-bytes-to-var"=520687618, "UART3-read-availabe-bytes"=520687632, "UART3-read-skip-bytes"=520163329, "UART3-read"=520097808, "UART3-read-Var"=520097810, "IO-read_bank0"=3489665024, "IO-write_bank0"=3489660929, "IO-read_bank1"=3506442240, "IO-write_bank1"=3506438145, "DA0-0_LED365"=2684354561, "DA0-1_LED385"=2685403137, "DA0-2_LED440"=2686451713, "DA0-3_LED470"=2687500289, "DA0-4_LED510"=2688548865, "DA0-5_LED550"=2689597441, "DA0-6_LED590"=2690646017, "DA0-7_LED640"=2691694593, "DA1-0_LED-R"=2701131777, "DA1-1_LED-G"=2702180353, "DA1-2_LED-B"=2703228929, "DA1-3_LED-AF"=2704277505, "DA1-4"=2705326081, "DA1-5"=2706374657, "DA1-6"=2707423233, "DA1-7"=2708471809, "DA2-Laser0"=2717908993, "DA2-Laser1"=2718957569, "DA2-Laser2"=2720006145, "DA2-Laser3"=2721054721, "DA2-Laser4"=2722103297, "Analog-read_AD0-0"=2818576384, "Analog-read-store_AD0-0"=2818572290, "AF-Register-transfer r/w"=2835349505, "AF-Register-read"=2835353600, "AF-Register-read-to-var"=2835353602, "AF-Transfer-from-var"=2835349507, "IO-delay_bank0"=3489923073, "IO-delay_bank0_fromVar"=3489923075, "read_cam_clock"=3289124864, "store_cam_clock"=3289120770, "read_cam_phase"=3289190400, "store_cam_phase"=3289186306, "store_cam_phase-t"=3289190402, "r_cam1_NHS"=3254980608, "w_cam1_NHS"=3254976513, "r_cam1_NVS"=3255046144, "w_cam1_NVS"=3255042049, "r_cam1_npx"=3255111680, "w_cam1_npx"=3255107585, "r_cam1_npy"=3255177216, "w_cam1_npy"=3255173121, "r_cam1_xhswait"=3255439360, "w_cam1_xhswait"=3255435265, "r_cam1_xvs_wait"=3255504896, "w_cam1_xvs_wait"=3255500801, "r_cam1_framcounter"=3255570432, "r_cam1_line"=3255635968, "r_cam1_xhs-counter"=3255701504, "r_cam2_NHS"=3271757824, "w_cam2_NHS"=3271753729, "r_cam2_NVS"=3271823360, "w_cam2_NVS"=3271819265, "r_cam2_npx"=3271888896, "w_cam2_npx"=3271884801, "r_cam2_npy"=3271954432, "w_cam2_npy"=3271950337, "r_cam2_xvs_wait"=3272282112, "w_cam2_xvs_wait"=3272278017, "r_cam2_framcounter"=3272347648, "r_cam2_line"=3272413184, "r_cam2_xhs-counter"=3272478720, "start TMSI"=102694919, "set_1Galvo"=101712113, "set_x-Galvo"=102760689, "set_y-Galvo"=103809265, "set_z-Fokus"=104857841, "set_1Galvo_position-only"=101711937, "set_x-Galvo_position-only"=102760513, "set_y-Galvo_position-only"=103809089, "set_z-Fokus_position-only"=104857665, "set_x-Galvo_position-only_ticket"=102764609, "set_y-Galvo_position-only_ticket"=103813185, "set_z-Fokus_position-only_ticket"=104861761, "set_1Galvo_relativ-only"=101712001, "set_x-Galvo_relativ-only"=102760577, "set_y-Galvo_relativ-only"=103809153, "set_z-Fokus_relativ-only"=104857729, "set_1Galvo_speed-only"=101711905, "set_x-Galvo_speed-only"=102760481, "set_y-Galvo_speed-only"=103809057, "set_z-Fokus_speed-only"=104857633, "set_1Galvo_acc-only"=101711889, "set_x-Galvo_acc-only"=102760465, "set_y-Galvo_acc-only"=103809041, "set_z-Fokus_acc-only"=104857617, "read_1Galvo_ticket"=101716032, "read_x-Galvo_ticket"=102764608, "read_y-Galvo_ticket"=103813184, "read_z-Focus_ticket"=104861760, "x-Galvo_pos_fromVar"=102760515, "y-Galvo_pos_fromVar"=103809091, "z-Focus_pos_fromVar"=104857667, "Servo0"=67108865, "Servo0-enable"=68091911, "Servo0-disable"=68091919, "Servo1"=68157441, "Servo1-enable"=69140487, "Servo1-disable"=69140495, "Servo2-enable"=70189063, "Servo2"=69206017, "Servo3-enable"=71237639, "Servo3"=70254593, "x-ssi-init"=202309639, "x-ssi-disable"=202309647, "x-ssi-Bits"=201523201, "x-ssi-Read"=201330688, "x-ssi-ReadToVar"=201326594, "x-ssi-ReadToVar-ticket"=201330690, "y-ssi-init"=203358215, "y-ssi-disable"=203358223, "y-ssi-Bits"=202571777, "y-ssi-Read"=202379264, "y-ssi-ReadToVar"=202375170, "y-ssi-ReadToVat-ticket"=202379266]; "P5-ticket" format="%.0x"; "P0" format="%.0x"; "P2" format="%.0x"; "P1" format="%.0x"}
  in  "TSM":T12={"RS232-axis"=255, "axis"=255, "Command"="?TILL_STATUS", "value"=946.0} {"RS232-axis" format="%0d"}
  in  "String":string(combo)="SOUR2:POW:LEV:IMM:AMPL?\r"
  in  "Wait ms":i32=500
  in  "direkt commands":T11(array[cluster])=[{"Delay 10µs"=0, "command"=102694919, "P0"=0, "P1"=0, "P2"=0, "P3"=0, "P4"=0, "P5-ticket"=0, "comment"=""}] {"command" format="%x" items=["end_no_ticket"=4027514895, "end_ticket"=4027518991, "NoOp"=4026531840, "Read ticks"=4026535936, "Read ticks to var"=4026535938, "Read IP"=4043313152, "Read IP into var"=4043313154, "Set IP from var"=4043309059, "Set IP from var, relative"=4043313155, "branchRel_if_equal"=4043374849, "decrement_branchRel_if_equal"=4043374945, "decrement_branchRel_if_greaterequal"=4043375201, "decrement_branchRel_if_greaterequal_withTicket"=4043379297, "decrement_branchRel_if_smaller"=4043375457, "increment_branchRel_if_smaller"=4043375473, "readVar"=4060090368, "writeVar"=4060086273, "copyVar0_from_var1"=4060086275, "math_addToVariable"=4076863488, "math_addVToVariable"=4076863489, "math_subToVariable"=4076863490, "math_subVToVariable"=4076863491, "math_multToVariable"=4076863492, "math_multvToVariable"=4076863493, "math_divideToVariable"=4076863494, "math_divideVToVariable"=4076863495, "math_modToVariable"=4076863496, "math_modVToVariable"=4076863497, "logic_and"=4093640704, "logic_or"=4093640706, "logic_xor"=4093640708, "bitshift"=4093640712, "I2C-write"=335544337, "I2C-read"=335548433, "Cam-SPI-write"=3254779905, "UART0-VC-Baud-write"=469958673, "UART0-VC-Baud-read"=469962768, "UART0-VC-write"=469762065, "UART0-VC-write-Var"=469762067, "UART0-VC-read-availabe-bytes-to-var"=470355970, "UART0-VC-read-availabe-bytes"=470355984, "UART0-VC-read-skip-bytes"=469831681, "UART0-VC-read"=469766160, "UART0-VC-read-Var"=469766162, "UART1-TSM-Baud-write"=486735889, "UART1-TSM-Baud-read"=486739984, "UART1-TSM-write"=486539281, "UART1-TSM-write-Var"=486539283, "UART1-TSM-read-availabe-bytes-to-var"=487133186, "UART1-TSM-read-availabe-bytes"=487133200, "UART1-TSM-read-skip-bytes"=486604801, "UART1-TSM-read-skip-bytes"=486608897, "UART1-TSM-read"=486543376, "UART1-TSM-read-Var"=486543378, "UART2-Laser-Baud-write"=503513105, "UART2-Baud-read"=503517200, "UART2-write"=503316497, "UART2-write-Var"=503316499, "UART2-read-availabe-bytes-to-var"=503910402, "UART2-read-availabe-bytes"=503910416, "UART2-read-skip-bytes"=503386113, "UART2-read"=503320592, "UART2-read-Var"=503320594, "UART3-Baud-write"=520290321, "UART3-Baud-read"=520294416, "UART3-write"=520093713, "UART3-write-Var"=520093715, "UART3-read-availabe-bytes-to-var"=520687618, "UART3-read-availabe-bytes"=520687632, "UART3-read-skip-bytes"=520163329, "UART3-read"=520097808, "UART3-read-Var"=520097810, "IO-read_bank0"=3489665024, "IO-write_bank0"=3489660929, "IO-read_bank1"=3506442240, "IO-write_bank1"=3506438145, "DA0-0_LED365"=2684354561, "DA0-1_LED385"=2685403137, "DA0-2_LED440"=2686451713, "DA0-3_LED470"=2687500289, "DA0-4_LED510"=2688548865, "DA0-5_LED550"=2689597441, "DA0-6_LED590"=2690646017, "DA0-7_LED640"=2691694593, "DA1-0_LED-R"=2701131777, "DA1-1_LED-G"=2702180353, "DA1-2_LED-B"=2703228929, "DA1-3_LED-AF"=2704277505, "DA1-4"=2705326081, "DA1-5"=2706374657, "DA1-6"=2707423233, "DA1-7"=2708471809, "DA2-Laser0"=2717908993, "DA2-Laser1"=2718957569, "DA2-Laser2"=2720006145, "DA2-Laser3"=2721054721, "DA2-Laser4"=2722103297, "Analog-read_AD0-0"=2818576384, "Analog-read-store_AD0-0"=2818572290, "AF-Register-transfer r/w"=2835349505, "AF-Register-read"=2835353600, "AF-Register-read-to-var"=2835353602, "AF-Transfer-from-var"=2835349507, "IO-delay_bank0"=3489923073, "IO-delay_bank0_fromVar"=3489923075, "read_cam_clock"=3289124864, "store_cam_clock"=3289120770, "read_cam_phase"=3289190400, "store_cam_phase"=3289186306, "store_cam_phase-t"=3289190402, "r_cam1_NHS"=3254980608, "w_cam1_NHS"=3254976513, "r_cam1_NVS"=3255046144, "w_cam1_NVS"=3255042049, "r_cam1_npx"=3255111680, "w_cam1_npx"=3255107585, "r_cam1_npy"=3255177216, "w_cam1_npy"=3255173121, "r_cam1_xhswait"=3255439360, "w_cam1_xhswait"=3255435265, "r_cam1_xvs_wait"=3255504896, "w_cam1_xvs_wait"=3255500801, "r_cam1_framcounter"=3255570432, "r_cam1_line"=3255635968, "r_cam1_xhs-counter"=3255701504, "r_cam2_NHS"=3271757824, "w_cam2_NHS"=3271753729, "r_cam2_NVS"=3271823360, "w_cam2_NVS"=3271819265, "r_cam2_npx"=3271888896, "w_cam2_npx"=3271884801, "r_cam2_npy"=3271954432, "w_cam2_npy"=3271950337, "r_cam2_xvs_wait"=3272282112, "w_cam2_xvs_wait"=3272278017, "r_cam2_framcounter"=3272347648, "r_cam2_line"=3272413184, "r_cam2_xhs-counter"=3272478720, "start TMSI"=102694919, "set_1Galvo"=101712113, "set_x-Galvo"=102760689, "set_y-Galvo"=103809265, "set_z-Fokus"=104857841, "set_1Galvo_position-only"=101711937, "set_x-Galvo_position-only"=102760513, "set_y-Galvo_position-only"=103809089, "set_z-Fokus_position-only"=104857665, "set_x-Galvo_position-only_ticket"=102764609, "set_y-Galvo_position-only_ticket"=103813185, "set_z-Fokus_position-only_ticket"=104861761, "set_1Galvo_relativ-only"=101712001, "set_x-Galvo_relativ-only"=102760577, "set_y-Galvo_relativ-only"=103809153, "set_z-Fokus_relativ-only"=104857729, "set_1Galvo_speed-only"=101711905, "set_x-Galvo_speed-only"=102760481, "set_y-Galvo_speed-only"=103809057, "set_z-Fokus_speed-only"=104857633, "set_1Galvo_acc-only"=101711889, "set_x-Galvo_acc-only"=102760465, "set_y-Galvo_acc-only"=103809041, "set_z-Fokus_acc-only"=104857617, "read_1Galvo_ticket"=101716032, "read_x-Galvo_ticket"=102764608, "read_y-Galvo_ticket"=103813184, "read_z-Focus_ticket"=104861760, "x-Galvo_pos_fromVar"=102760515, "y-Galvo_pos_fromVar"=103809091, "z-Focus_pos_fromVar"=104857667, "Servo0"=67108865, "Servo0-enable"=68091911, "Servo0-disable"=68091919, "Servo1"=68157441, "Servo1-enable"=69140487, "Servo1-disable"=69140495, "Servo2-enable"=70189063, "Servo2"=69206017, "Servo3-enable"=71237639, "Servo3"=70254593, "x-ssi-init"=202309639, "x-ssi-disable"=202309647, "x-ssi-Bits"=201523201, "x-ssi-Read"=201330688, "x-ssi-ReadToVar"=201326594, "x-ssi-ReadToVar-ticket"=201330690, "y-ssi-init"=203358215, "y-ssi-disable"=203358223, "y-ssi-Bits"=202571777, "y-ssi-Read"=202379264, "y-ssi-ReadToVar"=202375170, "y-ssi-ReadToVat-ticket"=202379266]; "P5-ticket" format="%.0x"; "P0" format="%.0x"; "P2" format="%.0x"; "P1" format="%.0x"}
  in  "ReturnBytes":u16=4
  out "init error":errorcluster
  in  "New Ini":bool
  in  "end-read":bool
  out "Return":i32[](array[numeric])=[120, 0] format="%.0x"
  out "send error":errorcluster
  out "recieve error":errorcluster
  out "Send debug":T11(array[cluster]) {"command" format="%x" items=["end_no_ticket"=4027514895, "end_ticket"=4027518991, "NoOp"=4026531840, "Read ticks"=4026535936, "Read ticks to var"=4026535938, "Read IP"=4043313152, "Read IP into var"=4043313154, "Set IP from var"=4043309059, "Set IP from var, relative"=4043313155, "branchRel_if_equal"=4043374849, "decrement_branchRel_if_equal"=4043374945, "decrement_branchRel_if_greaterequal"=4043375201, "decrement_branchRel_if_greaterequal_withTicket"=4043379297, "decrement_branchRel_if_smaller"=4043375457, "increment_branchRel_if_smaller"=4043375473, "readVar"=4060090368, "writeVar"=4060086273, "copyVar0_from_var1"=4060086275, "math_addToVariable"=4076863488, "math_addVToVariable"=4076863489, "math_subToVariable"=4076863490, "math_subVToVariable"=4076863491, "math_multToVariable"=4076863492, "math_multvToVariable"=4076863493, "math_divideToVariable"=4076863494, "math_divideVToVariable"=4076863495, "math_modToVariable"=4076863496, "math_modVToVariable"=4076863497, "logic_and"=4093640704, "logic_or"=4093640706, "logic_xor"=4093640708, "bitshift"=4093640712, "I2C-write"=335544337, "I2C-read"=335548433, "Cam-SPI-write"=3254779905, "UART0-VC-Baud-write"=469958673, "UART0-VC-Baud-read"=469962768, "UART0-VC-write"=469762065, "UART0-VC-write-Var"=469762067, "UART0-VC-read-availabe-bytes-to-var"=470355970, "UART0-VC-read-availabe-bytes"=470355984, "UART0-VC-read-skip-bytes"=469831681, "UART0-VC-read"=469766160, "UART0-VC-read-Var"=469766162, "UART1-TSM-Baud-write"=486735889, "UART1-TSM-Baud-read"=486739984, "UART1-TSM-write"=486539281, "UART1-TSM-write-Var"=486539283, "UART1-TSM-read-availabe-bytes-to-var"=487133186, "UART1-TSM-read-availabe-bytes"=487133200, "UART1-TSM-read-skip-bytes"=486604801, "UART1-TSM-read-skip-bytes"=486608897, "UART1-TSM-read"=486543376, "UART1-TSM-read-Var"=486543378, "UART2-Laser-Baud-write"=503513105, "UART2-Baud-read"=503517200, "UART2-write"=503316497, "UART2-write-Var"=503316499, "UART2-read-availabe-bytes-to-var"=503910402, "UART2-read-availabe-bytes"=503910416, "UART2-read-skip-bytes"=503386113, "UART2-read"=503320592, "UART2-read-Var"=503320594, "UART3-Baud-write"=520290321, "UART3-Baud-read"=520294416, "UART3-write"=520093713, "UART3-write-Var"=520093715, "UART3-read-availabe-bytes-to-var"=520687618, "UART3-read-availabe-bytes"=520687632, "UART3-read-skip-bytes"=520163329, "UART3-read"=520097808, "UART3-read-Var"=520097810, "IO-read_bank0"=3489665024, "IO-write_bank0"=3489660929, "IO-read_bank1"=3506442240, "IO-write_bank1"=3506438145, "DA0-0_LED365"=2684354561, "DA0-1_LED385"=2685403137, "DA0-2_LED440"=2686451713, "DA0-3_LED470"=2687500289, "DA0-4_LED510"=2688548865, "DA0-5_LED550"=2689597441, "DA0-6_LED590"=2690646017, "DA0-7_LED640"=2691694593, "DA1-0_LED-R"=2701131777, "DA1-1_LED-G"=2702180353, "DA1-2_LED-B"=2703228929, "DA1-3_LED-AF"=2704277505, "DA1-4"=2705326081, "DA1-5"=2706374657, "DA1-6"=2707423233, "DA1-7"=2708471809, "DA2-Laser0"=2717908993, "DA2-Laser1"=2718957569, "DA2-Laser2"=2720006145, "DA2-Laser3"=2721054721, "DA2-Laser4"=2722103297, "Analog-read_AD0-0"=2818576384, "Analog-read-store_AD0-0"=2818572290, "AF-Register-transfer r/w"=2835349505, "AF-Register-read"=2835353600, "AF-Register-read-to-var"=2835353602, "AF-Transfer-from-var"=2835349507, "IO-delay_bank0"=3489923073, "IO-delay_bank0_fromVar"=3489923075, "read_cam_clock"=3289124864, "store_cam_clock"=3289120770, "read_cam_phase"=3289190400, "store_cam_phase"=3289186306, "store_cam_phase-t"=3289190402, "r_cam1_NHS"=3254980608, "w_cam1_NHS"=3254976513, "r_cam1_NVS"=3255046144, "w_cam1_NVS"=3255042049, "r_cam1_npx"=3255111680, "w_cam1_npx"=3255107585, "r_cam1_npy"=3255177216, "w_cam1_npy"=3255173121, "r_cam1_xhswait"=3255439360, "w_cam1_xhswait"=3255435265, "r_cam1_xvs_wait"=3255504896, "w_cam1_xvs_wait"=3255500801, "r_cam1_framcounter"=3255570432, "r_cam1_line"=3255635968, "r_cam1_xhs-counter"=3255701504, "r_cam2_NHS"=3271757824, "w_cam2_NHS"=3271753729, "r_cam2_NVS"=3271823360, "w_cam2_NVS"=3271819265, "r_cam2_npx"=3271888896, "w_cam2_npx"=3271884801, "r_cam2_npy"=3271954432, "w_cam2_npy"=3271950337, "r_cam2_xvs_wait"=3272282112, "w_cam2_xvs_wait"=3272278017, "r_cam2_framcounter"=3272347648, "r_cam2_line"=3272413184, "r_cam2_xhs-counter"=3272478720, "start TMSI"=102694919, "set_1Galvo"=101712113, "set_x-Galvo"=102760689, "set_y-Galvo"=103809265, "set_z-Fokus"=104857841, "set_1Galvo_position-only"=101711937, "set_x-Galvo_position-only"=102760513, "set_y-Galvo_position-only"=103809089, "set_z-Fokus_position-only"=104857665, "set_x-Galvo_position-only_ticket"=102764609, "set_y-Galvo_position-only_ticket"=103813185, "set_z-Fokus_position-only_ticket"=104861761, "set_1Galvo_relativ-only"=101712001, "set_x-Galvo_relativ-only"=102760577, "set_y-Galvo_relativ-only"=103809153, "set_z-Fokus_relativ-only"=104857729, "set_1Galvo_speed-only"=101711905, "set_x-Galvo_speed-only"=102760481, "set_y-Galvo_speed-only"=103809057, "set_z-Fokus_speed-only"=104857633, "set_1Galvo_acc-only"=101711889, "set_x-Galvo_acc-only"=102760465, "set_y-Galvo_acc-only"=103809041, "set_z-Fokus_acc-only"=104857617, "read_1Galvo_ticket"=101716032, "read_x-Galvo_ticket"=102764608, "read_y-Galvo_ticket"=103813184, "read_z-Focus_ticket"=104861760, "x-Galvo_pos_fromVar"=102760515, "y-Galvo_pos_fromVar"=103809091, "z-Focus_pos_fromVar"=104857667, "Servo0"=67108865, "Servo0-enable"=68091911, "Servo0-disable"=68091919, "Servo1"=68157441, "Servo1-enable"=69140487, "Servo1-disable"=69140495, "Servo2-enable"=70189063, "Servo2"=69206017, "Servo3-enable"=71237639, "Servo3"=70254593, "x-ssi-init"=202309639, "x-ssi-disable"=202309647, "x-ssi-Bits"=201523201, "x-ssi-Read"=201330688, "x-ssi-ReadToVar"=201326594, "x-ssi-ReadToVar-ticket"=201330690, "y-ssi-init"=203358215, "y-ssi-disable"=203358223, "y-ssi-Bits"=202571777, "y-ssi-Read"=202379264, "y-ssi-ReadToVar"=202375170, "y-ssi-ReadToVat-ticket"=202379266]; "P5-ticket" format="%.0x"; "Delay 10µs" format="%.0x"; "P0" format="%.0x"; "P1" format="%.0x"}
  out "Ini-file used":path
  in  "wrapper[U32]":u32[](array[ring])=[67] format="%x" items=["p-Stop"=112, "1-ReInit FPGA"=49, "C-Clear Error"=67, "d-Dump registers"=100, "r-Read register"=114, "D-Dump memory"=68, "t-run"=116, "w-Write"=119]
  in  "Wrapper":bool
  in  "End":bool
  # "better this scales, for each device? - So far not implememted\ne.g Galvo +-30°opt,f=50mm: 7.9897E-7 m/count"
  # "ring has to match command!"
  # "HW=val*scale+offset  (also offset ist in hardwareunits)(time in v,a in s or 10µs units?)"
  # "scale    offset   min max maxa maxv  name"
  # "Version 5.2024 \nread digital \nnow ZMQ interface port 9912 9913\nworking: connect , reconnect"
  # "vielleicht automatisch je nach ticketbereich Codierung des Returns? Hex/Ascii..."
  # "Neu: Parabolic!"
  # "read cam: e.g. AC076=704630 \n(/256/100)=27.5246µs"
  # "alles umgestellt auf count und Pixel und 10µs !!!"
  # "shift full phase"
  # "PC timing"
  # "0: dcc22\n1: technosoft\n2: laser\n3: dc1000, usb,thermo\nTicket 0: response FIFO bytes"
  # "cr=\\r\nlf=\\n"
  # "16bit is shiftetd to msb (*65536)"
  # "todo: TSM other than UART1"
  # "MSR [6E81]: upd,Event,On,x/reached,contour,complete,trigger/LSN,LSP,wrap,x/err,SW,upd-Err,Init\nMER [0]: Off,CommErr,UV,OV, OT-d,OT-m,I2T,OC,LSN,LSP,Wrap,SerialE,ContE,Setup,short,CAN"
  # "version 20220216"
  # "cmd, err"
  # "logger for special tickets???"
  # "hex"
  # "77,2,30 > camtrigger"
  # "update values if exsiting"
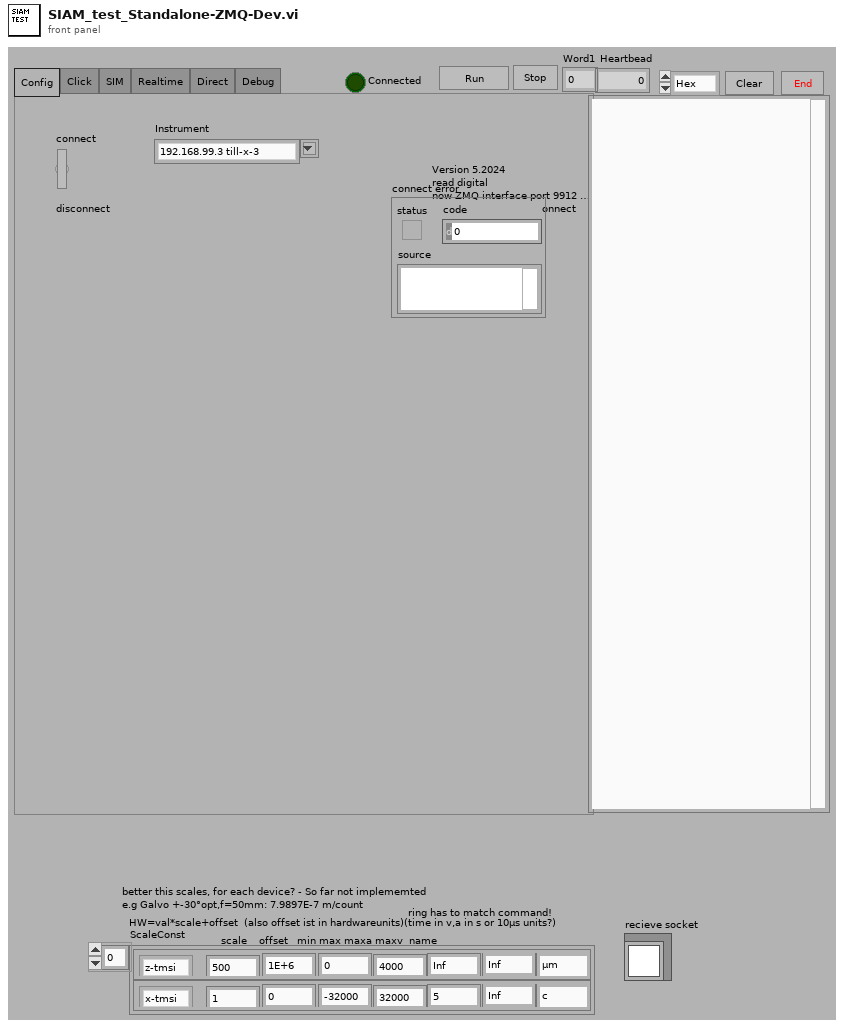
[diagram p1: front panel]
types:
  T1 = typedef "SIAM-axis.ctl" = u32
  T2 = cluster{"Axis-Ring":T1, "Scale":dbl, "Offset":dbl, "HW min":dbl, "HW max":dbl, "max a":dbl, "max v":dbl, "units":string}[]
  T3 = enum32{"Config", "Click", "SIM", "Realtime", "Direct", "Debug"}
  T4 = cluster{"Linear":cluster{"Axis-Ring":T1, "Position":i32}, "Linear":cluster{"Axis-Ring":T1, "Position":i32}, "Linear 2":cluster{"Axis-Ring":T1, "Position":i32}, "Linear 3":cluster{"Axis-Ring":T1, "Position":i32}, "Linear":cluster{"Axis-Ring":T1, "Position":i32}, "Linear 4":cluster{"Axis-Ring":T1, "Position":i32}, "Linear 5":cluster{"Axis-Ring":T1, "Position":i32}, "Linear 6":cluster{"Axis-Ring":T1, "Position":i32}, "Linear 7":cluster{"Axis-Ring":T1, "Position":i32}, "Linear 8":cluster{"Axis-Ring":T1, "Position":i32}, "Linear 9":cluster{"Axis-Ring":T1, "Position":i32}, "Linear 10":cluster{"Axis-Ring":T1, "Position":i32}, "Linear 11":cluster{"Axis-Ring":T1, "Position":i32}, "Linear 12":cluster{"Axis-Ring":T1, "Position":i32}, "Linear 13":cluster{"Axis-Ring":u32, "Position":i32}}
  T5 = cluster{"Digital-out":enum8{"cam1", "cam1-ready?", "cam2", "cam2-ready?", "tmsx?", "tsmy?", "tsm3?", "lid?", "led1", "led2", "led3", "led4", "led5", "led6", "led7", "led8", "durchR", "tsm-pwr", "dc-pwr", "laser-pwr", "Laser0", "Laser1", "Laser2", "Laser3", "Laser4", "LaserX", "TrigOut", "SMB1", ""}, "Boolean":bool}[]
  T6 = cluster{"x":bool, "y":bool, "-x":bool, "-y":bool}
  T7 = cluster{"Camera-Expos ms":dbl, "CameraImages":u16, "cam fps min.":dbl}
  T8 = typedef "SIAM_command.ctl" = u32
  T9 = cluster{"galvox-Line0":i16, "GalvoX-Blanking":dbl, "galvox-count/pix":dbl, "Camera-StartLine":i32, "Camera-Endline":u32, "Wobbel-total":dbl, "SM_ticks":u32, "Trigger_ticks":u32, "galvoxAccel":dbl, "WobbelAccel":dbl, "zAccel":dbl, "z-delay-ticks":u32, "SCMOS-LineSpeed [10µs]":dbl, "RS height- Pix":u16, "extra-xgalvo":dbl, "zcommand":T8, "min turn ticks":dbl}
  T10 = cluster{"z-distance_motorunits":i32, "#planes":u16, "Digital-out":enum8{"cam1", "cam1-ready?", "cam2", "cam2-ready?", "tmsx?", "tsmy?", "tsm3?", "lid?", "led1", "led2", "led3", "led4", "led5", "led6", "led7", "led8", "durchR", "durchG", "durchB", "AF", "Laser0", "Laser1", "Laser2", "Laser3", "Laser4", "LaserX", "TrigOut", "SMB1", ""}, "NoOfPhaseImages":u16}
  T11 = cluster{"Delay 10µs":u32, "command":T8, "P0":i32, "P1":i32, "P2":i32, "P3":i32, "P4":i32, "P5-ticket":i32, "comment":string}[]
  T12 = cluster{"RS232-axis":u8, "axis":u8, "Command":string, "value":dbl}
  T13 = typedef "zeromq.lvlib/socket_type.ctl" = enum8{"ZMQ_PAIR", "ZMQ_PUB", "ZMQ_SUB", "ZMQ_REQ", "ZMQ_REP", "ZMQ_DEALER", "ZMQ_ROUTER", "ZMQ_PULL", "ZMQ_PUSH", "ZMQ_XPUB", "ZMQ_XSUB", "ZMQ_STREAM", "ZMQ_SERVER", "ZMQ_CLIENT", "ZMQ_RADIO", "ZMQ_DISH", "ZMQ_GATHER", "ZMQ_SCATTER", "ZMQ_DGRAM"}
  T14 = typedef "zeromq.lvlib/socket_options.ctl" = enum8{"NONE", "ZMQ_HWM", "<2>", "ZMQ_SWAP", "ZMQ_AFFINITY", "ZMQ_ROUTING_ID", "ZMQ_SUBSCRIBE", "ZMQ_UNSUBSCRIBE", "ZMQ_RATE", "ZMQ_RECOVERY_IVL", "ZMQ_MCAST_LOOP", "ZMQ_SNDBUF", "ZMQ_RCVBUF", "ZMQ_RCVMORE", "ZMQ_FD", "ZMQ_EVENTS", "ZMQ_TYPE", "ZMQ_LINGER", "ZMQ_RECONNECT_IVL", "ZMQ_BACKLOG", "ZMQ_RECOVERY_IVL_MSEC", "ZMQ_RECONNECT_IVL_MAX", "ZMQ_MAXMSGSIZE", "ZMQ_SNDHWM", "ZMQ_RCVHWM", "ZMQ_MULTICAST_HOPS", "<26>", "ZMQ_RCVTIMEO", "ZMQ_SNDTIMEO", "<29>", "<30>", "ZMQ_IPV4ONLY", "ZMQ_LAST_ENDPOINT", "ZMQ_ROUTER_MANDATORY", "ZMQ_TCP_KEEPALIVE", "ZMQ_TCP_KEEPALIVE_CNT", "ZMQ_TCP_KEEPALIVE_IDLE", "ZMQ_TCP_KEEPALIVE_INTVL", "ZMQ_TCP_ACCEPT_FILTER", "ZMQ_IMMEDIATE", "ZMQ_XPUB_VERBOSE", "ZMQ_ROUTER_RAW", "ZMQ_IPV6", "ZMQ_MECHANISM", "ZMQ_PLAIN_SERVER", "ZMQ_PLAIN_USERNAME", "ZMQ_PLAIN_PASSWORD", "ZMQ_CURVE_SERVER", "ZMQ_CURVE_PUBLICKEY", "ZMQ_CURVE_SECRETKEY", "ZMQ_CURVE_SERVERKEY", "ZMQ_PROBE_ROUTER", "ZMQ_REQ_CORRELATE", "ZMQ_REQ_RELAXED", "ZMQ_CONFLATE", "ZMQ_ZAP_DOMAIN", "ZMQ_ROUTER_HANDOVER", "ZMQ_TOS", "ZMQ_IPC_FILTER_PID", "ZMQ_IPC_FILTER_UID", "ZMQ_IPC_FILTER_GID", "ZMQ_CONNECT_ROUTING_ID", "ZMQ_GSSAPI_SERVER", "ZMQ_GSSAPI_PRINCIPAL", "ZMQ_GSSAPI_SERVICE_PRINCIPAL", "ZMQ_GSSAPI_PLAINTEXT", "ZMQ_HANDSHAKE_IVL", "<67>", "ZMQ_SOCKS_PROXY", "ZMQ_XPUB_NODROP", "ZMQ_BLOCKY", "ZMQ_XPUB_MANUAL", "ZMQ_XPUB_WELCOME_MSG", "ZMQ_STREAM_NOTIFY", "ZMQ_INVERT_MATCHING", "ZMQ_HEARTBEAT_IVL", "ZMQ_HEARTBEAT_TTL", "ZMQ_HEARTBEAT_TIMEOUT", "ZMQ_XPUB_VERBOSER", "ZMQ_CONNECT_TIMEOUT", "ZMQ_TCP_MAXRT", "ZMQ_THREAD_SAFE", "<82>", "<83>", "ZMQ_MULTICAST_MAXTPDU", "ZMQ_VMCI_BUFFER_SIZE", "ZMQ_VMCI_BUFFER_MIN_SIZE", "ZMQ_VMCI_BUFFER_MAX_SIZE", "ZMQ_VMCI_CONNECT_TIMEOUT", "ZMQ_USE_FD", "ZMQ_GSSAPI_PRINCIPAL_NAMETYPE", "ZMQ_GSSAPI_SERVICE_PRINCIPAL_NAMETYPE", "ZMQ_BINDTODEVICE", "ZMQ_ZAP_ENFORCE_DOMAIN", "ZMQ_LOOPBACK_FASTPATH", "ZMQ_METADATA", "ZMQ_MULTICAST_LOOP", "ZMQ_ROUTER_NOTIFY"}
  T15 = cluster{"Delay 10µs":u32, "command":T8, "P0":i32, "P1":i32, "P2":i32, "P3":i32, "P4":i32, "P5-ticket":i32, string}[]
  T16 = cluster{"rel 10µs":u32, "Device":T8, "data0":i32, "data1":i32, "data2":i32, "data3":i32, "data4":i32, "data5":i32, string}
  T17 = cluster{"Delay 10µs":u32, "command":T8, "P0":i32, "P1":i32, "P2":i32, "P3":i32, "P4":i32, "P5-ticket":i32, "comment":string}
  T18 = enum8{"cam1", "cam1-ready?", "cam2", "cam2-ready?", "tmsx?", "tsmy?", "tsm3?", "lid?", "led1", "led2", "led3", "led4", "led5", "led6", "led7", "led8", "durchR", "tsm-pwr", "dc-pwr", "laser-pwr", "Laser0", "Laser1", "Laser2", "Laser3", "Laser4", "LaserX", "TrigOut", "SMB1", ""}
  T19 = cluster{"rel 10µs":u32, "Device":T8, "data0":i32, "data1":i32, "data2":i32, "data3":i32, "data4":i32, "data5":i32, string}[]
  T20 = cluster{"Delay 10µs":u32, "command":T8, "P0":i32, "P1":i32, "P2":i32, "P3":i32, "P4":i32, "P5-ticket":i32, "Comment":string}[]
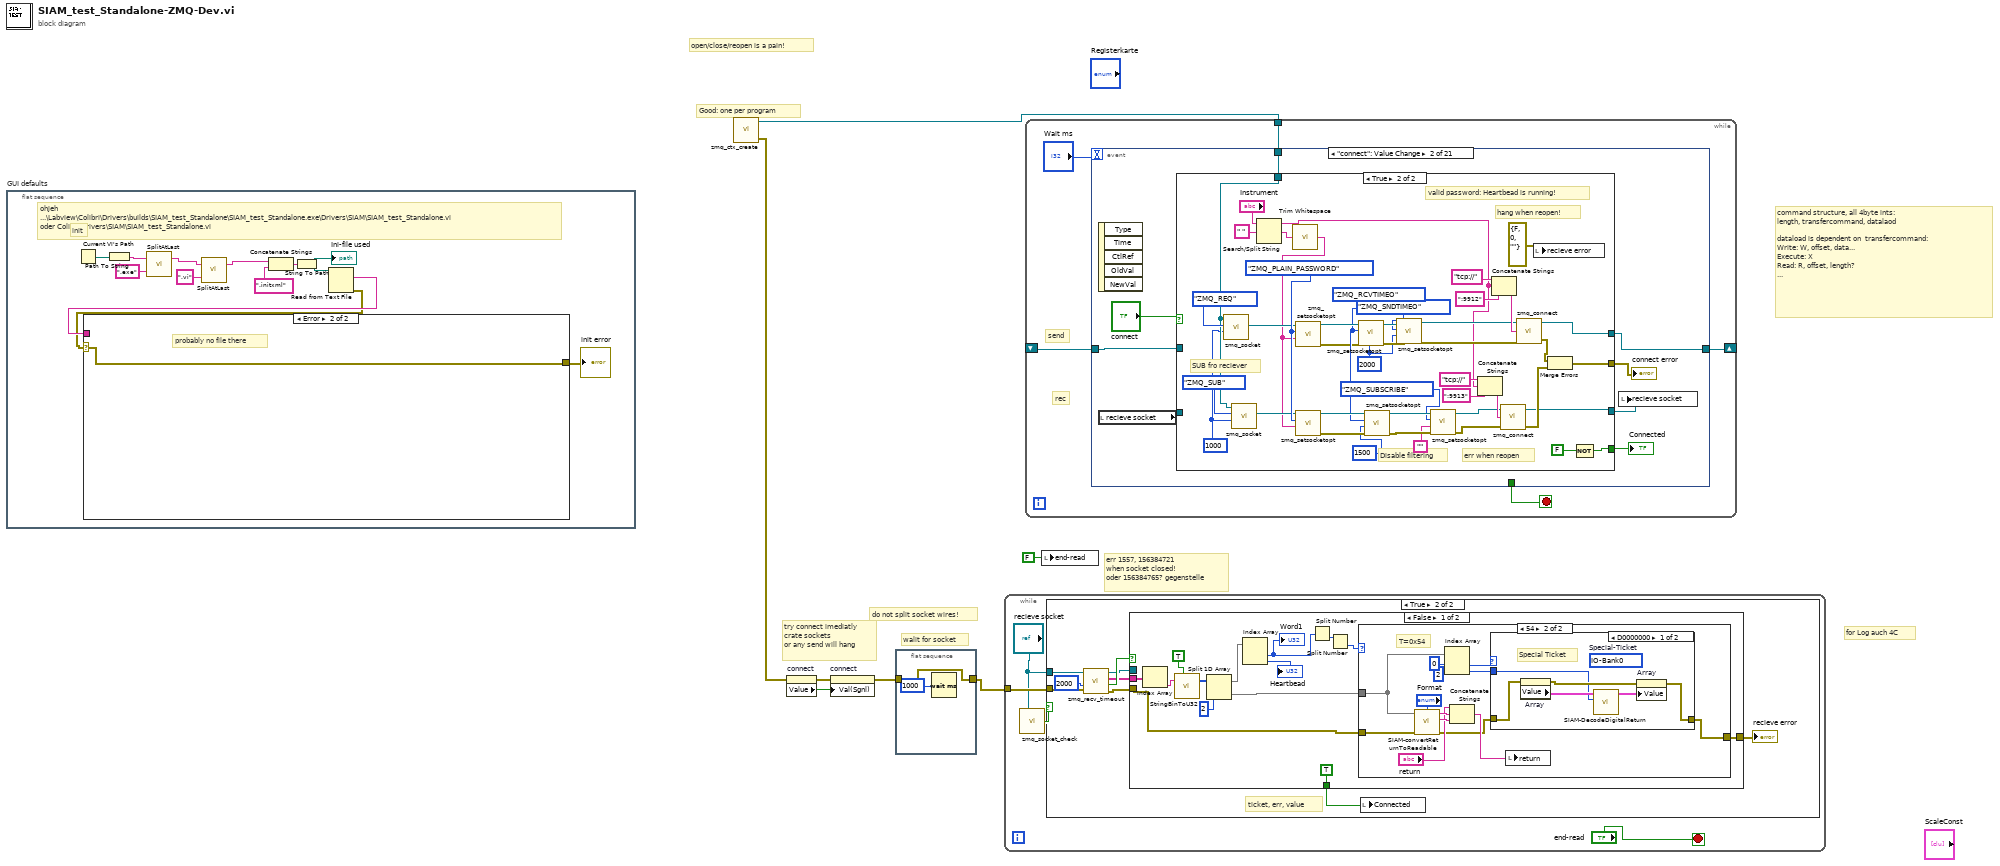
[diagram p0: block diagram]
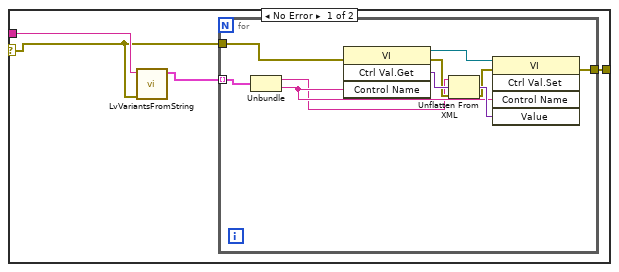
[diagram p2: hidden frame]
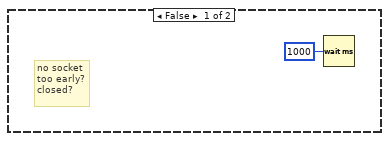
[diagram p3: hidden frame]
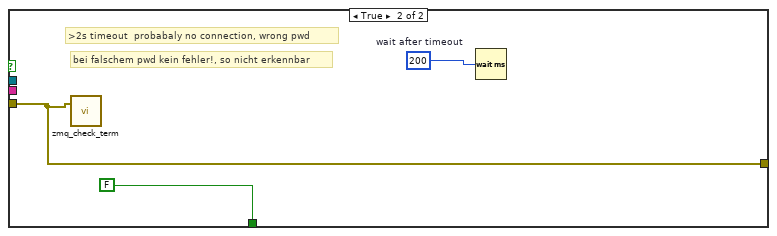
[diagram p6: hidden frame]
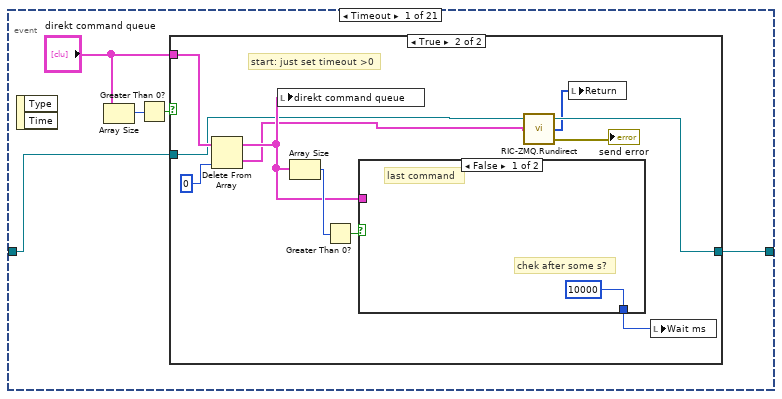
[diagram p7: hidden frame]
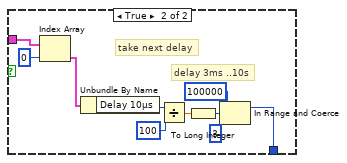
[diagram p9: hidden frame]
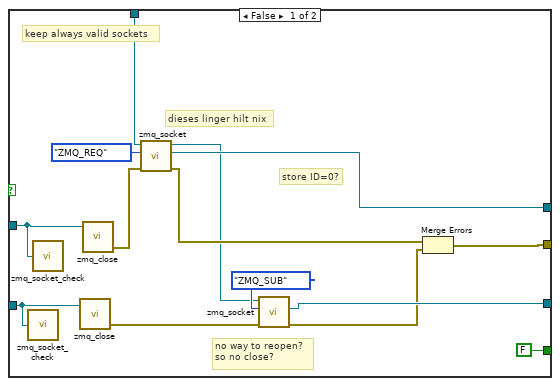
[diagram p10: hidden frame]
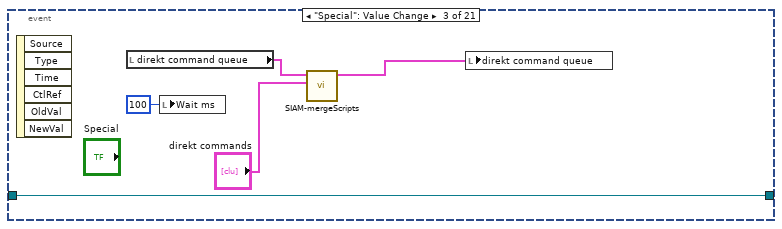
[diagram p11: hidden frame]
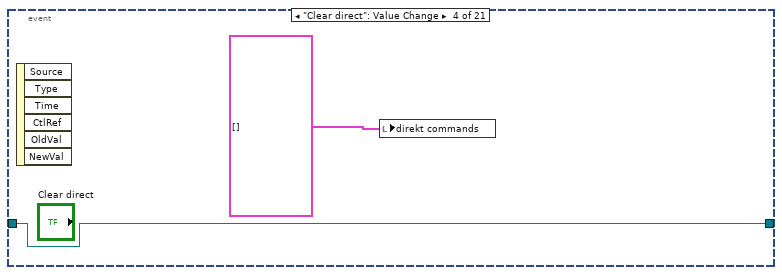
[diagram p12: hidden frame]
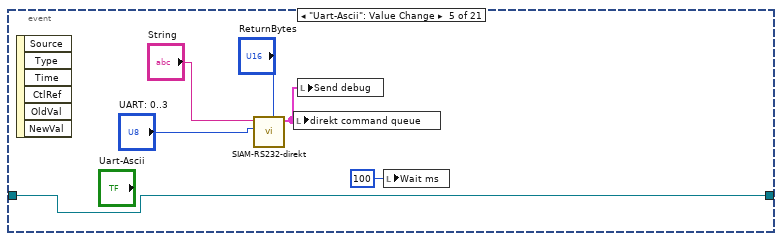
[diagram p13: hidden frame]
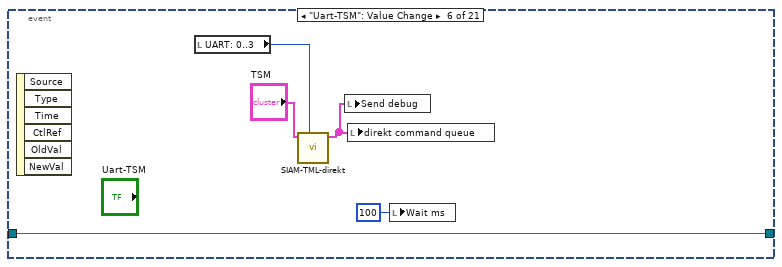
[diagram p14: hidden frame]
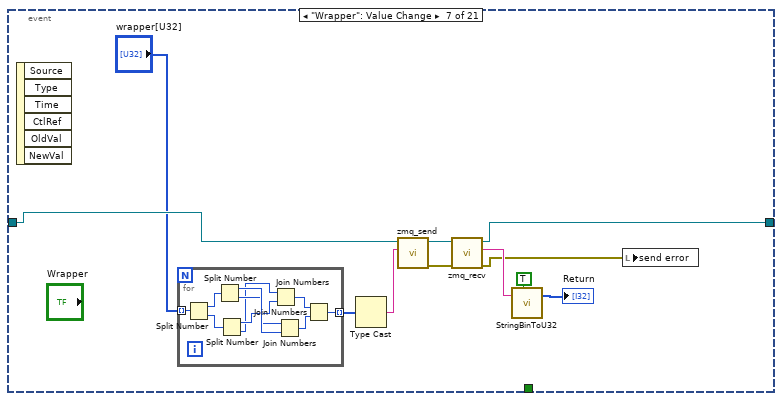
[diagram p15: hidden frame]
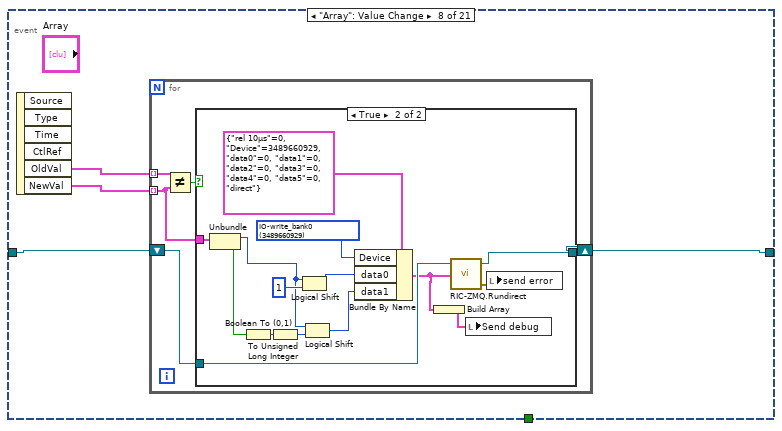
[diagram p16: hidden frame]
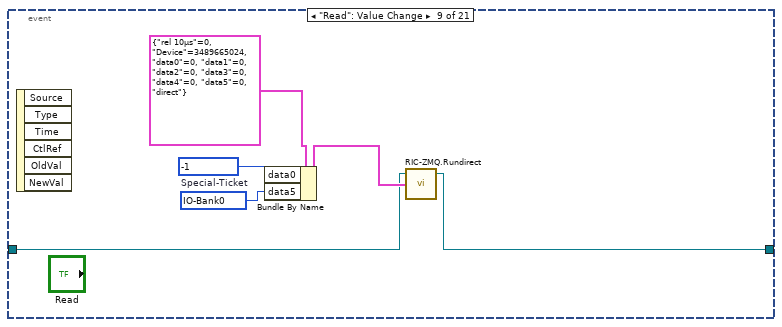
[diagram p18: hidden frame]
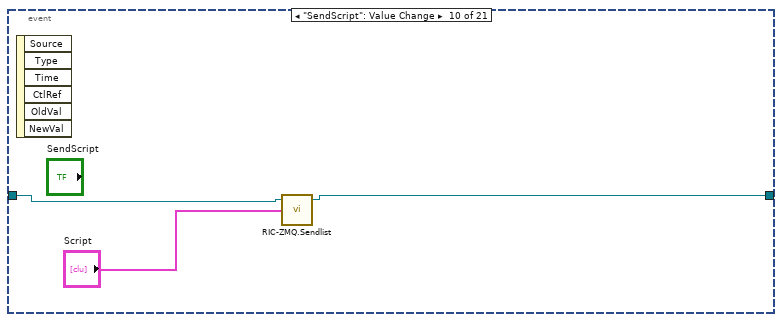
[diagram p19: hidden frame]
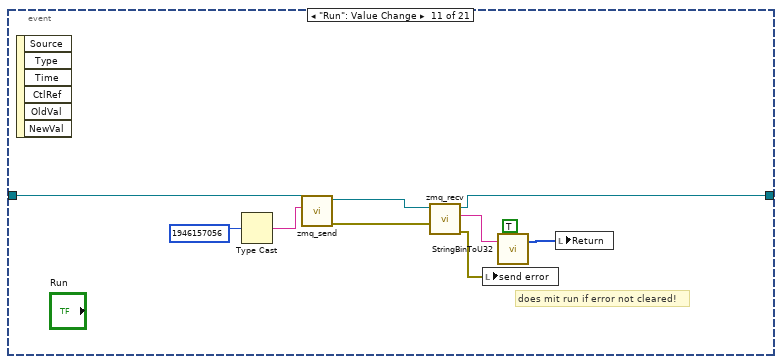
[diagram p20: hidden frame]
diagram:
  # "for Log auch 4C"
  # "walit for socket"
  # "err 1557, 156384721\nwhen socket closed!\noder 156384765? gegenstelle"
  # "open/close/reopen is a pain!"
  # "try connect imediatly\ncrate sockets \nor any send will hang"
  # "do not split socket wires!"
  # "Good: one per program"
  # "command structure, all 4byte ints:\nlength, transfercommand, datalaod\n\ndataload is dependent on  transfercommand:\nWrite: W, offset, data...\nExecute: X\nRead: R, offset, length?\n..."
  n1 = flat-sequence "GUI defaults" {
    frame #0 {
      # "ohjeh\n...\\Labview\\Colibri\\Drivers\\builds\\SIAM_test_Standalone\\SIAM_test_Standalone.exe\\Drivers\\SIAM\\SIAM_test_Standalone.vi\noder Colibri\\Drivers\\SIAM\\SIAM_test_Standalone.vi"
      # "init"
      n2 = Current VI's Path() -> (path=w11:path)
      n3 = Path To String(path=w11) -> (string=w14:string)
      n4 = call "SplitAtLast.vi"("search char"=".exe", "In-String"=w14) -> ("Front (default)"=w10:string)  [unwired: 1 out]
      n5 = call "SplitAtLast.vi"("search char"=".vi", "In-String"=w10) -> ("Front (default)"=w9:string)  [unwired: 1 out]
      n6 = Concatenate Strings(w9, ".initxml" ("string")) -> (w13:string)
      n7 = String To Path(string=w13) -> (path=w12:path)
      "Ini-file used" <- w12
      n8 = Read from Text File(file (use dialog)=w12) -> (text=w18:string, error out=w17:errorcluster)  [unwired: 3 in, 2 out]
      n9 = case shown="Error" w17 {
        selector: w17 -> [w21 w34]
        tunnel: w18 -> [w22 _]
        tunnel: [w23 w34] -> w16
        frame No Error {
          n10 = call "LvVariantsFromString.vi"("error IO"=w21, "iniString"=w22) -> ("Array"=w20:cluster{"LvVariant":string, "Name":string}[])  [unwired: 8 in, 1 out]
          n11 = for {
            tunnel: w21 -> [w33]
            tunnel: [w27] -> w23
            tunnel: w20 -> [w26] mode=indexing
            n12 = Unbundle(w26) -> ("LvVariant"=w24:string, "Name"=w25:string)
            n13 = invoke class="VI" method="Ctrl Val.Get"(error in=w33, "Control Name"=w25) -> (reference out=w32:refnum<vi>, error out=w29:errorcluster, "Get Control Value Variant"=w31:variant)  [unwired: 2 in, 1 out]
            n14 = Unflatten From XML(xml string=w24, type=w31, error in (no error)=w29) -> (value=w30:variant, error out=w28:errorcluster)
            n15 = invoke class="VI" method="Ctrl Val.Set"(reference=w32, error in=w28, "Control Name"=w25, "Value"=w30) -> (error out=w27:errorcluster)  [unwired: 1 in, 4 out]
          }
        }
        frame Error {
          # "probably no file there"
        }
      }
      "init error" <- w16
    }
  }
  n16 = call "zmq_ctx_create.vi"() -> ("error out"=w3:errorcluster, "context out"=w6:refnum<class "zmq_context.lvclass">)  [unwired: 4 in]
  n17 = property on="connect" class="Bool (strict)"(error in=w3) -> (error out=w5:errorcluster, "Value"=w4:bool)  [unwired: 1 in, 1 out]
  n18 = property on="connect" class="Bool (strict)"(error in=w5, "Val(Sgnl)"=w4) -> (error out=w2:errorcluster)  [unwired: 1 in, 1 out]
  n19 = flat-sequence {
    tunnel: w2 -> [w35]
    tunnel: [w35] -> w1
    frame #0 {
      n20 = Wait (ms)(milliseconds to wait=u32 1000) -> ()  [unwired: 1 out]
    }
  }
  n21 = while {
    tunnel: w1 -> [w39]
    stop <- "end-read" stop-if-true
    n22 = call "zmq_socket_check.vi"("socket in"="recieve socket") -> ("valid?"=w37:bool)
    n23 = case shown="True" w37 {
      tunnel: w39 -> [_ w49]
      tunnel: "recieve socket" -> [_ w42]
      frame False {
        # "no socket\ntoo early?\nclosed?"
        n24 = Wait (ms)(milliseconds to wait=u32 1000) -> ()  [unwired: 1 out]
      }
      frame True {
        # "ticket, err, value"
        n25 = call "zmq_recv_timeout.vi"("error in"=w49, "timeout (ms)"=u32 2000, "socket in"=w42) -> ("error out"=w47:errorcluster, "timeout?"=w48:bool, "parts"=w44:string[], "socket out"=w45:refnum<class "zmq_socket.lvclass">)  [unwired: 1 in]
        n26 = case shown="False" w48 {
          tunnel: [w53 w86] -> w50
          tunnel: w47 -> [w52 w86]
          tunnel: w45 -> [_ _]
          tunnel: w44 -> [w55 _]
          tunnel: [TRUE ("Connected") FALSE ("Connected")] -> w43
          frame False {
            n27 = Index Array(array=w55) -> (element=w54:string)  [unwired: 1 in]
            n28 = call "StringBinToU32.vi"("String"=w54, "Swap Byte order"=TRUE) -> ("Array"=w63:i32[])  [unwired: 3 in]
            n29 = Split 1D Array(array=w63, index=2) -> (first subarray=w60:i32[], second subarray=w59:i32[])
            n30 = Index Array(array=w60) -> (element #1=w58:i32, element #2=→"Heartbead":i32)  [unwired: 2 in]
            "Word1" <- w58
            n31 = Split Number(x=w58) -> (lo(x)=w57:u16)  [unwired: 1 out]
            n32 = Split Number(x=w57) -> (lo(x)=w56:u8)  [unwired: 1 out]
            n33 = case shown="54" w56 {
              tunnel: [w65 w70] -> w53
              tunnel: w59 -> [_ w67]
              tunnel: w52 -> [w65 w66]
              frame 0, Default {
                # "H heartbead\nL: Log"
              }
              frame 84 {
                # "T=0x54"
                n34 = call "SIAM-convertReturnToReadable.vi"("Format"="Format", "error in (no error)"=w66, "Return"=w67) -> ("error out"=w71:errorcluster, "CR?"=w76:string, "Readable"=w77:string)  [unwired: 6 out]
                n35 = Index Array(array=w67, index #1=0 ("index"), index #2=2 ("index")) -> (element #1=w73:i32, element #2=w68:i32)
                n36 = Concatenate Strings("return", w77, w76) -> (w78:string)
                n37 = case shown="D0000000" w73 {
                  tunnel: w71 -> [w84 w85]
                  tunnel: [w82 w85] -> w70
                  tunnel: w68 -> [w80 _]
                  frame -805306368 {
                    (unwired) T1 3489660928 items=["255Axis"=16777217, "1-Axis"=17825793, "2-Axis"=18874369, "3-Axis"=19922945, "4-Axis"=20971521, "5-Axis"=22020097, "6-Axis"=23068673, "7-Axis"=24117249, "LED365"=2684354561, "LED385"=2685403137, "LED440"=2686451713, "LED470"=2687500289, "LED510"=2688548865, "LED540"=2689597441, "LED590"=2690646017, "LED640"=2691694593, "DurchR"=2701131777, "DurchG"=2702180353, "DurchB"=2703228929, "AF"=2704277505, "Laser0"=2717908993, "Laser1"=2718957569, "Laser2"=2720006145, "Laser3"=2721054721, "Servo0"=67108865, "Servo1"=68157441, "Servo2"=69206017, "Servo3"=70254593, "0-TMSI"=100663361, "1-TMSI"=101711937, "x-tmsi"=102760513, "y-tmsi"=103809089, "z-tmsi"=104857665, "orca1"=503316481, "orca2"=503316482, "orca3"=503316483, "orca4"=503316484, "IO-Bank0"=3489660928, "IO-Bank1"=3506438144, ""=0]  # Special-Ticket
                    # "Special Ticket"
                    n38 = property on="Array" class="Arr (strict)"(error in=w84) -> (error out=w83:errorcluster, "Value"=w81:T5)  [unwired: 1 in, 1 out]
                    n39 = call "SIAM-DecodeDigitalReturn.vi"(10:w80, "Array 2"=w81) -> ("Array 3"=w79:T5)  [unwired: 9 in]
                    n40 = property on="Array" class="Arr (strict)"(error in=w83, "Value"=w79) -> (error out=w82:errorcluster)  [unwired: 1 in, 1 out]
                  }
                  frame 0, Default {
                  }
                }
                n41 = local write "return"(w78) -> ()
              }
            }
          }
          frame True {
            w88 = u32 200  # wait after timeout
            # "bei falschem pwd kein fehler!, so nicht erkennbar"
            # ">2s timeout  probabaly no connection, wrong pwd"
            n42 = call "zmq_check_term.vi"("error in"=w86) -> ()  [unwired: 1 in, 2 out]
            n43 = Wait (ms)(milliseconds to wait=w88) -> ()  [unwired: 1 out]
          }
        }
        "recieve error" <- w50
        n44 = local write "Connected"(w43) -> ()
      }
    }
  }
  n45 = while {
    shift-right: [w90] -> _
    shift-left: _ -> [w91]
    tunnel: w6 -> [w89]
    stop <- w93 stop-if-true
    # "rec"
    # "send"
    n46 = event shown="[1] \"connect\": Value Change" {
      selector: _ -> [_ _ _ _ _ _ _ _ _ _ _ _ _ _ _ _ _ _ _ _ _]
      dyn-events: _ -> [_ _ _ _ _ _ _ _ _ _ _ _ _ _ _ _ _ _ _ _ _]
      timeout: "Wait ms" -> [_ _ _ _ _ _ _ _ _ _ _ _ _ _ _ _ _ _ _ _ _]
      tunnel: [_ _ _ _ _ _ _ _ _ _ _ _ _ _ _ _ _ _ _ _ "End"] -> w93
      tunnel: w91 -> [w95 w127 w188 w193 w197 w202 w211 w228 w253 w260 w266 w275 w280 w283 w290 w295 w314 w353 w356 w358 w388]
      tunnel: [w94 w126 w188 w193 w197 w202 w207 w227 w252 w258 w263 w274 w280 w283 w290 w295 w314 w353 w356 w358 w388] -> w90
      tunnel: w89 -> [_ w125 _ _ _ _ _ _ _ _ _ _ _ _ _ _ _ _ _ _ w385]
      event Timeout {
        n47 = event-data() -> ()  [unwired: 3 out]
        n48 = Array Size(array="direkt command queue") -> (size(s)=w97:i32)
        n49 = Greater Than 0?(x=w97) -> (x > 0?=w96:bool)
        n50 = case shown="True" w96 {
          tunnel: "direkt command queue" -> [_ w108]
          tunnel: w95 -> [w99 w104]
          tunnel: [w99 w101] -> w94
          frame False {
            # "no command queued"
          }
          frame True {
            # "start: just set timeout >0"
            n51 = Delete From Array(array=w108, index=0) -> (deleted portion=w103:T17, array with subset deleted=w105:T11)  [unwired: 1 in]
            n52 = local write "direkt command queue"(w105) -> ()
            n53 = Array Size(array=w105) -> (size(s)=w107:i32)
            n54 = Greater Than 0?(x=w107) -> (x > 0?=w106:bool)
            n55 = case shown="False" w106 {
              tunnel: [10000 ("upper limit") w121] -> w110
              tunnel: w105 -> [_ w120]
              frame False {
                # "chek after some s?"
                # "last command"
              }
              frame True {
                # "delay 3ms ..10s"
                # "take next delay"
                n56 = Index Array(array=w120, index=0) -> (element=w113:T17)
                n57 = Unbundle By Name(w113) -> ("Delay 10µs"=w119:u32)
                n58 = Divide(x=w119, y=u32 100) -> (x/y=w117:dbl)
                n59 = To Long Integer(number=w117) -> (32bit integer=w114:i32)
                n60 = In Range and Coerce(upper limit=100000, x=w114, lower limit=3) -> (coerced(x)=w121:i32)  [unwired: 1 out]
              }
            }
            n61 = call "RIC-ZMQ.Rundirect.vi"("socket in"=w104, "Cluster"=w103) -> ("socket out"=w101:refnum<class "zmq_socket.lvclass">, "Return"=w100:i32[], "error out"=→"send error":errorcluster)  [unwired: 2 in, 1 out]
            n62 = local write "Return"(w100) -> ()
            n63 = local write "Wait ms"(w110) -> ()
          }
        }
      }
      event "connect": Value Change {
        n64 = event-data() -> ()  [unwired: 6 out]
        n65 = local read "recieve socket"() -> (w124:refnum<class "zmq_socket.lvclass">)
        n66 = case shown="True" "connect" {
          tunnel: [FALSE w186] -> w128
          tunnel: w124 -> [w130 _]
          tunnel: w127 -> [w131 _]
          tunnel: [w142 w177] -> w126
          tunnel: w125 -> [w139 w158]
          tunnel: [w137 w151] -> w123
          tunnel: [w136 w149] -> w122
          frame False {
            # "keep always valid sockets"
            # "dieses linger hilt nix"
            # "no way to reopen?\nso no close?"
            # "store ID=0?"
            n67 = call "zmq_socket_check.vi"("socket in"=w130) -> ()  [unwired: 1 out]
            n68 = call "zmq_socket_check.vi"("socket in"=w131) -> ()  [unwired: 1 out]
            n69 = call "zmq_close.vi"("socket"=w130) -> ("error out"=w135:errorcluster)  [unwired: 4 in]
            n70 = call "zmq_close.vi"("socket"=w131) -> ("error out"=w140:errorcluster)  [unwired: 4 in]
            n71 = call "zmq_socket.vi"("error in"=w140, "socket type"=socket_type."ZMQ_REQ", "context in"=w139) -> ("error out"=w133:errorcluster, "socket out"=w142:refnum<class "zmq_socket.lvclass">, "context out"=w132:refnum<class "zmq_context.lvclass">)  [unwired: 2 in]
            n72 = call "zmq_socket.vi"("error in"=w135, "socket type"=socket_type."ZMQ_SUB", "context in"=w132) -> ("error out"=w134:errorcluster, "socket out"=w137:refnum<class "zmq_socket.lvclass">)  [unwired: 2 in, 1 out]
            n73 = Merge Errors(w133, w134) -> (w136:errorcluster)
          }
          frame True {
            w150 = 1000 ("linger (ms)")
            w173 = 2000
            w168 = socket_options."ZMQ_RCVTIMEO" ("option")
            w179 = socket_options."ZMQ_PLAIN_PASSWORD" ("option")
            # "Disable filtering"
            # "SUB fro reciever"
            # "err when reopen"
            # "hang when reopen!"
            # "valid password: Heartbead is running!"
            n74 = call "zmq_socket.vi"("linger (ms)"=w150, "socket type"=socket_type."ZMQ_REQ", "context in"=w158) -> ("socket out"=w165:refnum<class "zmq_socket.lvclass">)  [unwired: 2 in, 2 out]
            n75 = call "zmq_socket.vi"("linger (ms)"=w150, "socket type"=socket_type."ZMQ_SUB", "context in"=w158) -> ("socket out"=w159:refnum<class "zmq_socket.lvclass">)  [unwired: 2 in, 2 out]
            n76 = Search/Split String(string="Instrument", search string/char (-)=" ") -> (substring before match=w144:string, match + rest of string=w148:string)  [unwired: 1 in, 1 out]
            n77 = call <vilib>:"Trim Whitespace.vi"("string"=w148) -> ("trimmed string"=w145:string)  [unwired: 1 in]
            n78 = call "zmq_setsocketopt.vi"("value"=w145, "option"=w179, "socket in"=w165) -> ("error out"=w166:errorcluster, "socket out"=w172:refnum<class "zmq_socket.lvclass">)  [unwired: 3 in]
            n79 = call "zmq_setsocketopt.vi"("value"=w145, "option"=w179, "socket in"=w159) -> ("error out"=w169:errorcluster, "socket out"=w170:refnum<class "zmq_socket.lvclass">)  [unwired: 3 in]
            n80 = call "zmq_setsocketopt.vi"("error in"=w166, "value"=w173, "option"=w168, "socket in"=w172) -> ("error out"=w175:errorcluster, "socket out"=w176:refnum<class "zmq_socket.lvclass">)  [unwired: 2 in]
            n81 = call "zmq_setsocketopt.vi"("error in"=w169, "value"=1500, "option"=w168, "socket in"=w170) -> ("error out"=w157:errorcluster, "socket out"=w154:refnum<class "zmq_socket.lvclass">)  [unwired: 2 in]
            n82 = call "zmq_setsocketopt.vi"("error in"=w175, "value"=w173, "option"=socket_options."ZMQ_SNDTIMEO", "socket in"=w176) -> ("error out"=w164:errorcluster, "socket out"=w171:refnum<class "zmq_socket.lvclass">)  [unwired: 2 in]
            n83 = call "zmq_setsocketopt.vi"("error in"=w157, "value"="", "option"=socket_options."ZMQ_SUBSCRIBE", "socket in"=w154) -> ("error out"=w156:errorcluster, "socket out"=w155:refnum<class "zmq_socket.lvclass">)  [unwired: 2 in]
            n84 = Concatenate Strings("tcp://" ("string"), w144, ":9913" ("string")) -> (w183:string)
            n85 = Concatenate Strings("tcp://" ("string"), w144, ":9912" ("string")) -> (w180:string)
            n86 = call "zmq_connect.vi"("error in"=w156, "endpoint"=w183, "socket in"=w155) -> ("error out"=w162:errorcluster, "socket out"=w151:refnum<class "zmq_socket.lvclass">)  [unwired: 1 in]
            n87 = call "zmq_connect.vi"("error in"=w164, "endpoint"=w180, "socket in"=w171) -> ("error out"=w163:errorcluster, "socket out"=w177:refnum<class "zmq_socket.lvclass">)  [unwired: 1 in]
            n88 = local write "recieve error"(errorcluster {"status"=FALSE, "code"=0, "source"=""} ("recieve error")) -> ()
            n89 = Merge Errors(w163, w162) -> (w149:errorcluster)
            n90 = Not(x=FALSE) -> (.not. x?=w186:bool)
          }
        }
        "Connected" <- w128
        "connect error" <- w122
        n91 = local write "recieve socket"(w123) -> ()
      }
      event "Special": Value Change {
        n92 = event-data() -> ()  [unwired: 7 out]
        n93 = local read "direkt command queue"() -> (w190:T11)
        n94 = local write "Wait ms"(100 ("Wait for")) -> ()
        n95 = call "SIAM-mergeScripts.vi"("Script 2"="direkt commands", "Script"=w190) -> ("Script out"=w189:T11)  [unwired: 8 in, 1 out]
        n96 = local write "direkt command queue"(w189) -> ()
      }
      event "Clear direct": Value Change {
        n97 = event-data() -> ()  [unwired: 7 out]
        n98 = local write "direkt commands"(T15 [] ("direkt commands")) -> ()
      }
      event "Uart-Ascii": Value Change {
        n99 = event-data() -> ()  [unwired: 7 out]
        n100 = call "SIAM-RS232-direkt.vi"("ReturnBytes"="ReturnBytes", "UART: 0..3"="UART: 0..3", "Combo Box"="String") -> ("Script"=w196:T11)  [unwired: 6 in, 2 out]
        n101 = local write "direkt command queue"(w196) -> ()
        n102 = local write "Send debug"(w196) -> ()
        n103 = local write "Wait ms"(100 ("Wait for")) -> ()
      }
      event "Uart-TSM": Value Change {
        n104 = event-data() -> ()  [unwired: 7 out]
        n105 = local read "UART: 0..3"() -> (w203:u8)
        n106 = call "SIAM-TML-direkt.vi"("UART: 0..3"=w203, "TSM"="TSM") -> ("Array"=w201:T11)  [unwired: 6 in, 3 out]
        n107 = local write "Send debug"(w201) -> ()
        n108 = local write "direkt command queue"(w201) -> ()
        n109 = local write "Wait ms"(100 ("Wait for")) -> ()
      }
      event "Wrapper": Value Change {
        n110 = event-data() -> ()  [unwired: 7 out]
        n111 = for {
          tunnel: "wrapper[U32]" -> [w226] mode=indexing
          tunnel: [w225] -> w210 mode=indexing
          n112 = Split Number(x=w226) -> (hi(x)=w224:u16, lo(x)=w223:u16)
          n113 = Split Number(x=w224) -> (hi(x)=w222:u8, lo(x)=w219:u8)
          n114 = Split Number(x=w223) -> (hi(x)=w218:u8, lo(x)=w217:u8)
          n115 = Join Numbers(hi=w217, lo=w218) -> ((hi.lo)=w220:u16)
          n116 = Join Numbers(hi=w219, lo=w222) -> ((hi.lo)=w221:u16)
          n117 = Join Numbers(hi=w220, lo=w221) -> ((hi.lo)=w225:u32)
        }
        n118 = Type Cast(x=w210) -> (*(type *) &x=w209:string)  [unwired: 1 out]
        n119 = call "zmq_send.vi"("data"=w209, "socket in"=w211) -> ("error out"=w212:errorcluster, "socket out"=w216:refnum<class "zmq_socket.lvclass">)  [unwired: 5 in]
        n120 = call "zmq_recv.vi"("error in"=w212, "socket in"=w216) -> ("error out"=w213:errorcluster, "data"=w214:string, "socket out"=w207:refnum<class "zmq_socket.lvclass">)  [unwired: 3 in, 2 out]
        n121 = call "StringBinToU32.vi"("String"=w214, "Swap Byte order"=TRUE) -> ("Array"=→"Return":i32[])  [unwired: 3 in]
        n122 = local write "send error"(w213) -> ()
      }
      event "Array": Value Change {
        n123 = event-data() -> ("OldVal"=w230:T5, "NewVal"=w229:T5)  [unwired: 5 out]
        n124 = for {
          tunnel: w230 -> [w235] mode=indexing
          tunnel: w229 -> [w233] mode=indexing
          shift-right: [w231] -> w227
          shift-left: w228 -> [w232]
          n125 = Not Equal?(x=w235, y=w233) -> (x != y?=w234:bool)
          n126 = case shown="True" w234 {
            tunnel: w233 -> [_ w244]
            tunnel: w232 -> [w236 w241]
            tunnel: [w236 w237] -> w231
            frame False {
            }
            frame True {
              w246 = T8 3489660929 items=["read_x-Motor_status_ticket"=17305600, "init_x-Motor"=17760263, "read_x-Motor_absolute_ticket"=16781312, "move_x-Motor_absolute"=16777217, "move_x-Motor_relative"=16842753, "read_y-Motor_status_ticket"=18354176, "init_y-Motor"=18808839, "read_y-Motor_absolute_ticket"=17829888, "move_y-Motor_absolute"=17825793, "move_y-Motor_relative"=17891329, "read_z-Motor_status_ticket"=19402752, "init_z-Motor"=19857415, "stop_z-Motor"=19857423, "start_z-Motor"=19857422, "read_z-Motor_absolute_ticket"=18878464, "move_z-Motor_absolute"=18874369, "move_z-Motor_relative"=18939905, "read_Objective_status_ticket"=20451328, "init_Objective"=20905991, "read_Objective_absolute_ticket"=19927040, "move_Objective_absolute"=19922945, "move_Objective_relative"=19988481, "read_Filter_status_ticket"=21499904, "init_Filter"=21954567, "read_Filter_absolute_ticket"=20975616, "move_Filter_absolute"=20971521, "move_Filter_relative"=21037057, "read_Trans-Rad_status_ticket"=22548480, "init_Trans-Rad"=23003143, "read_Trans-Rad_absolute_ticket"=22024192, "move_Trans-Rad_absolute"=22020097, "move_Trans-Rad_relative"=22085633, "read_FRET_status_ticket"=23597056, "init_FRET"=24051719, "read_FRET_absolute_ticket"=23072768, "move_FRET_absolute"=23068673, "move_FRET_relative"=23134209, "read_SI-Rad_status_ticket"=24645632, "init_SI-Rad"=25100295, "read_SI-Rad_absolute_ticket"=24121344, "move_SI-Rad_absolute"=24117249, "move_SI-Rad_relative"=24182785, "end_no_ticket"=4027514895, "end_ticket"=4027518991, "IO-read_bank0"=3489665024, "IO-write_bank0"=3489660929, "IO-read_bank1"=3506442240, "IO-write_bank1"=3506438145, "Analog-write_DA0-0"=2684354561, "Analog-write_DA0-1"=2685403137, "Analog-write_DA0-2"=2686451713, "Analog-write_DA0-3"=2687500289, "Analog-write_DA0-4"=2688548865, "Analog-write_DA0-5"=2689597441, "Analog-write_DA0-6"=2690646017, "Analog-write_DA0-7"=2691694593, "Analog-write_DA1-0"=2701131777, "Analog-write_DA1-1"=2702180353, "Analog-write_DA1-2"=2703228929, "Analog-write_DA1-3"=2704277505, "Analog-write_DA1-4"=2705326081, "Analog-write_DA1-5"=2706374657, "Analog-write_DA1-6"=2707423233, "Analog-write_DA1-7"=2708471809, "Analog-read_AD0-0"=2818576384, "Analog-read-store_AD0-0"=2818572290, "IO-delay_bank0"=3489923073, "IO-delay_bank0_fromVar"=3489923075, "read_cam_clock"=3289124864, "store_cam_clock"=3289120770, "read_cam_phase"=3289190400, "set_cam_deadtime"=3288989697, "set_cam_10uscycles"=3289055233, "set_cam_10uscycles_fromVariable"=3289055235, "calc_cam"=3289317386, "store_cam_Var"=3289251842, "math_addToVariable"=4060086278, "readVar"=4060090368, "writeVar"=4060086273, "copyVar"=4060086276, "decrement_branchRel_if_equal"=4043374945, "decrement_branchRel_if_greaterequal"=4043375201, "decrement_branchRel_if_greaterequal_withTicket"=4043379297, "decrement_branchRel_if_smaller"=4043375457, "increment_branchRel_if_smaller"=4043375473, "set_1Galvo"=101712113, "set_x-Galvo"=102760689, "set_y-Galvo"=103809265, "set_z-Fokus"=104857841, "set_1Galvo_position-only"=101711937, "set_x-Galvo_position-only"=102760513, "set_y-Galvo_position-only"=103809089, "set_z-Fokus_position-only"=104857665, "set_x-Galvo_position-only_ticket"=102764609, "set_y-Galvo_position-only_ticket"=103813185, "set_z-Fokus_position-only_ticket"=104861761, "set_x-Galvo_relativ-only"=102760577, "set_y-Galvo_relativ-only"=103809153, "set_z-Fokus_relativ-only"=104857729, "set_x-Galvo_speed-only"=102760481, "set_y-Galvo_speed-only"=103809057, "set_z-Fokus_speed-only"=104857633, "read_1Galvo_ticket"=101716032, "read_x-Galvo_ticket"=102764608, "read_y-Galvo_ticket"=103813184, "read_z-Focus_ticket"=104861760, "x-Galvo_pos_fromVar"=102760515, "y-Galvo_pos_fromVar"=103809091, "z-Focus_pos_fromVar"=104857667, "Servo0"=67108865, "Servo1"=68157441, "Servo2"=69206017] ("Device")
              n127 = Unbundle(w244) -> ("Digital-out"=w243:T18, "Boolean"=w242:bool)
              n128 = Boolean To (0,1)(Boolean=w242) -> (0, 1=w249:i16)
              n129 = To Unsigned Long Integer(number=w249) -> (unsigned 32bit integer=w245:u32)
              n130 = Logical Shift(y=w243, x=u32 1) -> (x << y=w248:u32)
              n131 = Logical Shift(y=w243, x=w245) -> (x << y=w247:u32)
              n132 = Bundle By Name(cluster=T16 {"rel 10µs"=0, "Device"=3489660929, "data0"=0, "data1"=0, "data2"=0, "data3"=0, "data4"=0, "data5"=0, "direct"} ("output cluster"), "Device"=w246, "data0"=w248, "data1"=w247) -> (w239:T16)
              n133 = Build Array(w239) -> (w238:T19)
              n134 = call "RIC-ZMQ.Rundirect.vi"("socket in"=w241, "Cluster"=w239) -> ("socket out"=w237:refnum<class "zmq_socket.lvclass">, "error out"=w240:errorcluster)  [unwired: 2 in, 2 out]
              n135 = local write "Send debug"(w238) -> ()
              n136 = local write "send error"(w240) -> ()
            }
          }
        }
      }
      event "Read": Value Change {
        w256 = T1 3489660928 items=["255Axis"=16777217, "1-Axis"=17825793, "2-Axis"=18874369, "3-Axis"=19922945, "4-Axis"=20971521, "5-Axis"=22020097, "6-Axis"=23068673, "7-Axis"=24117249, "LED365"=2684354561, "LED385"=2685403137, "LED440"=2686451713, "LED470"=2687500289, "LED510"=2688548865, "LED540"=2689597441, "LED590"=2690646017, "LED640"=2691694593, "DurchR"=2701131777, "DurchG"=2702180353, "DurchB"=2703228929, "AF"=2704277505, "Laser0"=2717908993, "Laser1"=2718957569, "Laser2"=2720006145, "Laser3"=2721054721, "Servo0"=67108865, "Servo1"=68157441, "Servo2"=69206017, "Servo3"=70254593, "0-TMSI"=100663361, "1-TMSI"=101711937, "x-tmsi"=102760513, "y-tmsi"=103809089, "z-tmsi"=104857665, "orca1"=503316481, "orca2"=503316482, "orca3"=503316483, "orca4"=503316484, "IO-Bank0"=3489660928, "IO-Bank1"=3506438144, ""=0]  # Special-Ticket
        n137 = event-data() -> ()  [unwired: 7 out]
        n138 = Bundle By Name(cluster=T16 {"rel 10µs"=0, "Device"=3489665024, "data0"=0, "data1"=0, "data2"=0, "data3"=0, "data4"=0, "data5"=0, "direct"} ("output cluster"), "data0"=-1, "data5"=w256) -> (w254:T16)
        n139 = call "RIC-ZMQ.Rundirect.vi"("socket in"=w253, "Cluster"=w254) -> ("socket out"=w252:refnum<class "zmq_socket.lvclass">)  [unwired: 2 in, 3 out]
      }
      event "SendScript": Value Change {
        n140 = event-data() -> ()  [unwired: 7 out]
        n141 = call "RIC-ZMQ.Sendlist.vi"("socket in"=w260, "Script"="Script") -> ("socket out"=w258:refnum<class "zmq_socket.lvclass">)  [unwired: 2 in, 3 out]
      }
      event "Run": Value Change {
        # "does mit run if error not cleared!"
        n142 = event-data() -> ()  [unwired: 7 out]
        n143 = Type Cast(x=1946157056) -> (*(type *) &x=w264:string)  [unwired: 1 out]
        n144 = call "zmq_send.vi"("data"=w264, "socket in"=w266) -> ("error out"=w270:errorcluster, "socket out"=w269:refnum<class "zmq_socket.lvclass">)  [unwired: 5 in]
        n145 = call "zmq_recv.vi"("error in"=w270, "socket in"=w269) -> ("error out"=w261:errorcluster, "data"=w267:string, "socket out"=w263:refnum<class "zmq_socket.lvclass">)  [unwired: 3 in, 2 out]
        n146 = local write "send error"(w261) -> ()
        n147 = call "StringBinToU32.vi"("String"=w267, "Swap Byte order"=TRUE) -> ("Array"=w262:i32[])  [unwired: 3 in]
        n148 = local write "Return"(w262) -> ()
      }
      event "Stop": Value Change {
        w272 = "p\u0000\u0000\u0000"  # Stop p
        n149 = event-data() -> ()  [unwired: 7 out]
        n150 = call "zmq_send.vi"("data"=w272, "socket in"=w275) -> ("error out"=w276:errorcluster, "socket out"=w279:refnum<class "zmq_socket.lvclass">)  [unwired: 5 in]
        n151 = call "zmq_recv.vi"("error in"=w276, "socket in"=w279) -> ("error out"=w271:errorcluster, "data"=w277:string, "socket out"=w274:refnum<class "zmq_socket.lvclass">)  [unwired: 3 in, 2 out]
        n152 = local write "send error"(w271) -> ()
        n153 = call "StringBinToU32.vi"("String"=w277, "Swap Byte order"=TRUE) -> ("Array"=w273:i32[])  [unwired: 3 in]
        n154 = local write "Return"(w273) -> ()
      }
      event "Save": Value Change {
        n155 = event-data() -> ()  [unwired: 7 out]
        n156 = local read "Script"() -> (w282:T11)
        n157 = call "SIAMScript_to_String.vi"("Script"=w282) -> ("String"=w281:string)  [unwired: 9 in, 1 out]
        n158 = Write to Text File(text=w281) -> ()  [unwired: 3 in, 3 out]
      }
      event "Load": Value Change {
        n159 = event-data() -> ()  [unwired: 7 out]
        n160 = Read from Text File(prompt (Open existing file)="Select File") -> (text=w285:string, error out=w284:errorcluster)  [unwired: 3 in, 2 out]
        n161 = case shown="No Error" w284 {
          selector: w284 -> [w287 _]
          tunnel: w285 -> [w288 _]
          frame No Error {
            n162 = call "ImportSIAMScript.vi"("error in (no error)"=w287, "String"=w288) -> ("Script"=w289:T20)  [unwired: 8 in, 1 out]
            n163 = local write "Script"(w289) -> ()
          }
          frame Error {
          }
        }
      }
      event "Calculate SIM": Value Change {
        n164 = event-data() -> ()  [unwired: 7 out]
        n165 = call "SIAM-SIMStack_v3.vi"("Constants"="Constants", "User"="User") -> ("SIAMScript"=w294:T11, "Camera"=→"Camera":T7)  [unwired: 7 in, 1 out]
        n166 = local write "Script"(w294) -> ()
      }
      event "Axis": Value Change {
        # "block frontpanel!"
        n167 = event-data() -> ("OldVal"=w299:T4, "NewVal"=w298:T4)  [unwired: 5 out]
        n168 = Cluster To Array(cluster=w299) -> (array=w296:cluster{"Axis-Ring":T1, "Position":i32}[])
        n169 = Cluster To Array(cluster=w298) -> (array=w297:cluster{"Axis-Ring":T1, "Position":i32}[])
        n170 = for {
          tunnel: w296 -> [w303] mode=indexing
          tunnel: w297 -> [w302] mode=indexing
          n171 = Not Equal?(x=w303, y=w302) -> (x != y?=w301:bool)
          n172 = case shown="True" w301 {
            tunnel: w302 -> [_ w313]
            frame False {
            }
            frame True {
              # "sorry direct too fast\nwork with Direkt list?"
              n173 = local read "direkt command queue"() -> (w307:T11)
              n174 = local read "TSM"() -> (w310:T12)
              n175 = Unbundle(w313) -> ("Axis-Ring"=w312:T1, "Position"=w311:i32)
              n176 = Unbundle By Name(w310) -> ("RS232-axis"=w309:u8)
              n177 = call "Axis-To-SIAM-direkt.vi"("Extra Information"=w309, "Position"=w311, "Axis-Ring"=w312) -> ("Direct Commands"=w306:T11)  [unwired: 7 in, 1 out]
              "Send debug" <- w306
              n178 = call "SIAM-mergeScripts.vi"("Enum"=enum16{"Append", "try merge"}."Append", "Script 2"=w306, "Script"=w307) -> ("Script out"=w305:T11)  [unwired: 7 in, 1 out]
              n179 = local write "direkt command queue"(w305) -> ()
              n180 = local write "Wait ms"(10 ("Wait ms")) -> ()
            }
          }
        }
        n181 = Wait (ms)(milliseconds to wait=u32 100) -> ()  [unwired: 1 out]
      }
      event "New Ini": Value Change {
        # "flatten to string"
        n182 = event-data() -> ()  [unwired: 7 out]
        n183 = Current VI's Path() -> (path=w326:path)
        n184 = Path To String(path=w326) -> (string=w328:string)
        n185 = call "SplitAtLast.vi"("search char"=".exe", "In-String"=w328) -> ("Front (default)"=w324:string)  [unwired: 1 out]
        n186 = call "SplitAtLast.vi"("search char"=".vi", "In-String"=w324) -> ("Front (default)"=w323:string)  [unwired: 1 out]
        n187 = Concatenate Strings(w323, ".initxml" ("string")) -> (w327:string)
        n188 = String To Path(string=w327) -> (path=w315:path)
        n189 = Read from Text File(file (use dialog)=w315) -> (refnum out=w317:refnum<file>, text=w321:string, error out=w322:errorcluster)  [unwired: 3 in, 1 out]
        n190 = case shown="Error" w322 {
          selector: w322 -> [w337 _]
          tunnel: w321 -> [w341 _]
          tunnel: [w338 w348] -> w320
          tunnel: [w336 w347] -> w316
          frame No Error {
            # "update existing entries"
            n191 = call "LvVariantsFromString.vi"("error IO"=w337, "iniString"=w341) -> ("error out"=w339:errorcluster, "Array"=w340:cluster{"LvVariant":string, "Name":string}[])  [unwired: 8 in]
            n192 = for {
              tunnel: w340 -> [w346] mode=indexing
              tunnel: w339 -> [w344]
              tunnel: [w343] -> w338 mode=indexing
              tunnel: [w342] -> w336
              # "ignore errors!"
              n193 = Unbundle(w346) -> ("Name"=w345:string)  [unwired: 1 out]
              n194 = invoke class="VI" method="Ctrl Val.Get"(error in=w344, "Control Name"=w345) -> (error out=w342:errorcluster, "Get Control Value Variant"=w343:variant)  [unwired: 2 in, 2 out]
            }
          }
          frame Error {
            # "all new"
            n195 = invoke class="VI" method="Ctrl Val.Get All"("Controls"=TRUE) -> (error out=w347:errorcluster, "Get All Control Values Variant"=w349:cluster{"Name":string, "Variant Data":variant}[])  [unwired: 3 in, 2 out]
            n196 = for {
              tunnel: w349 -> [w352] mode=indexing
              tunnel: [w351] -> w348 mode=indexing
              n197 = Unbundle By Name(w352) -> ("Variant Data"=w351:variant)
            }
          }
        }
        n198 = Close File(refnum=w317) -> ()  [unwired: 1 in, 2 out]
        n199 = local write "init error"(w316) -> ()
        n200 = for {
          shift-right: [w332] -> w318
          shift-left: "" -> [w335]
          tunnel: w320 -> [w331] mode=indexing
          n201 = Flatten To XML(anything=w331) -> (xml string=w334:string)
          n202 = Concatenate Strings(w335, w334, "\r\n") -> (w332:string)
        }
        n203 = Write to Text File(file (use dialog)=w315, text=w318) -> ()  [unwired: 2 in, 3 out]
      }
      event "Clear": Value Change {
        n204 = event-data() -> ()  [unwired: 7 out]
        n205 = case shown="False" "Clear" {
          frame False {
          }
          frame True {
            n206 = local write "return"("") -> ()
          }
        }
      }
      event "ClearScript": Value Change {
        n207 = event-data() -> ()  [unwired: 7 out]
        n208 = local write "Script"(T15 [] ("Script")) -> ()
      }
      event "xy": Value Change {
        n209 = event-data() -> ("OldVal"=w371:T6, "NewVal"=w370:T6)  [unwired: 5 out]
        n210 = Not Equal?(x=w371, y=w370) -> (x != y?=w369:T6)
        n211 = property on="Axis" class="Clust (strict)"() -> ("Value"=w361:T4)  [unwired: 2 in, 2 out]
        n212 = Unbundle(w369) -> ("x"=w368:bool, "-x"=w365:bool, "-y"=w366:bool)  [unwired: 1 out]
        n213 = Or(x=w365, y=w366) -> (x .or. y?=w364:bool)
        n214 = Or(x=w368, y=w365) -> (x .or. y?=w367:bool)
        n215 = Negate(x="step") -> (-x=w362:i32)
        n216 = Select(t=w362, s=w364, f="step") -> (s? t:f=w360:i32)
        n217 = case shown="True" w367 {
          tunnel: [w375 w379] -> w359
          tunnel: w361 -> [w374 w380]
          tunnel: w360 -> [w376 w381]
          frame False {
            # "y"
            n218 = Unbundle By Name(w374) -> ("Linear.Position"=w373:i32)
            n219 = Add(x=w373, y=w376) -> (x+y=w372:i32)
            n220 = Bundle By Name(cluster=w374, "Linear.Position"=w372) -> (w375:T4)
          }
          frame True {
            # "x"
            n221 = Unbundle By Name(w380) -> ("Linear.Position"=w378:i32)
            n222 = Add(x=w378, y=w381) -> (x+y=w377:i32)
            n223 = Bundle By Name(cluster=w380, "Linear.Position"=w377) -> (w379:T4)
          }
        }
        n224 = property on="Axis" class="Clust (strict)"("Val(Sgnl)"=w359) -> ()  [unwired: 2 in, 2 out]
      }
      event "End": Value Change {
        # "Clean up"
        n225 = event-data() -> ()  [unwired: 7 out]
        n226 = local read "recieve socket"() -> (w387:refnum<class "zmq_socket.lvclass">)
        n227 = call "zmq_close.vi"("socket"=w388) -> ("error out"=w386:errorcluster)  [unwired: 4 in]
        n228 = call "zmq_close.vi"("error in"=w386, "socket"=w387) -> ("error out"=w384:errorcluster)  [unwired: 3 in]
        n229 = call "zmq_ctx_destroy.vi"("error in"=w384, "reap? (F)"=TRUE, "context in"=w385) -> ("error out"=w382:errorcluster)  [unwired: 2 in]
        n230 = local write "connect error"(w382) -> ()
        n231 = local write "Connected"(FALSE ("Connected")) -> ()
        n232 = disable-structure shown="Disabled" {
          frame Disabled {
            n233 = invoke class="VI" method="FP.Close"() -> ()  [unwired: 3 in, 3 out]
          }
          frame Enabled {
          }
        }
        n234 = local write "end-read"("End") -> ()
      }
    }
  }
  n235 = local write "end-read"(FALSE ("end-read")) -> ()
